vi "Preference_Panel.vi"(0 "Mode":T1) -> ()   [LabVIEW 2010]
uses:
  Anemometry Sub Vis/Controls/Server_Comms.ctl
  Anemometry Sub Vis/Controls/Preference_Mode.ctl
  Anemometry Sub Vis/Controls/Overhead.ctl
  <vilib>/Instr/_visa.llb/VISA Find Search Mode.ctl
  ADAM Client/Sub VIs/ADAM Controls/Calib_type_ADAM.ctl
  ADAM Client/Sub VIs/ADAM Controls/Module_type_ADAM.ctl
  ADAM Client/Sub VIs/ADAM Controls/Ch_description_ADAM.ctl
  ADAM Client/Sub VIs/ADAM Controls/Function_ADAM.ctl
  ADAM Client/Sub VIs/ADAM Controls/Channel_State.ctl
  ADAM Client/Sub VIs/ADAM Controls/Address.ctl
  Anemometry Sub Vis/Globals/Constants_global.vi
  Anemometry Sub Vis/Globals/Preference_global.vi
  Anemometry Sub Vis/Globals/Trav_pos_global.vi
  Anemometry Sub Vis/Globals/Qnet_Globals.vi
  Anemometry Sub Vis/Acquisition/PWA/PWAtasksGLOBAL.vi
  Anemometry Sub Vis/Globals/Dynamic_call_global.ph.vi
panel:
  in  "Post Processing Machine":bool
  in  "Analogue Device Serial No.":string="1188AB4"
  in  "PWA Device Serial No.":string="1187C98"
  in  "ADAM Setup File":u16(ring) items=["Current_Setup.xls"]
  in  "Default Source Establishment Time (s)":dbl=20.0
  out "This Machine's IP Number":string
  in  "Rig Setup":u16(ring) items=["3_x_2_tunnel", "A_Tunnel", "Adam_Sayer_Desk", "ADAM_Server", "Aero_Tunnel", "Alex_Desktop", "B_Tunnel", "Calibration_Tunnel", "Contact_Conductance", "D_Tunnel", "EnFlo_Tunnel", "Frauke_Desktop", "iMac_G5_2", "iMacDuo1", "Matteo's_desktop", "Matteo_PC", "Nick_PC-2", "Paul_Desk-Paul_Desk_Machine", "Paul_Hayden-Desk", "Paul_N_Desk_Machine_2", "Post_Processing_Machine", "PowerBook_G4_1", "PowerBook_G4_2", "Syn_jet_rig", "Tank", "tdf", "Tom_Desk", "Towing_tank", "--New Rig Setup--"]
  in  "Default Traverse Name":u16(ring) items=["A_Tunnel", "Aero_ThroughWall", "Aero_Tunnel", "Angle_Calibrator", "B_Tunnel", "D_Tunnel", "Dummy_Traverse", "EnFlo_Stack", "EnFlo_Tunnel", "EnFlo_Turntable", "Laser_Meas_Traverse", "mohd_setup", "Paul_Desk_Test", "PIV_Traverse", "--New Traverse Setup--"]
  in  "OK":bool
  in  "% Error From First Calib":dbl=10.0 format="%.1f"
  in  "% Error From Previous Calib":dbl=0.5 format="%.1f"
  in  "Qnet Site Root":path=path "/G4_2_HD/Users/paulhayden/Qnet/qnet"
  out "Templates":path=path "/G4_2_HD/Applications (Mac OS 9)/EnFlo Software/Anemometry/Anemometry Sub Vis/Templates"
  in  "Data Folder":path
  out "EnFlo SW Preferences":path=path "/G4_2_HD/Applications (Mac OS 9)/LabVIEW 5.1/EnFlo SW Preferences"
  in  "Tunnel Speed Control":bool
  in  "SMTP server IP address":string
  in  "Abs Press (mbar)":string="Froude:NPL:Atmos_Press"
  in  "Temperature":string="EnFlo Tun:Inlet Heater:Av Temp"
  in  "Server port number":u32=3363
  in  "Server address":string
  in  "LabVIEW Administrators":string[](array[string])=["", "", "", "", "", "", "", "", "", "", "", "", "", "", "", "", "", "", "", ""]
  in  "Server Comms":T2=enum."Do Not Link To Server"
  # "Server Computer Peferences"
  # "Multi Run Preferences"
  # "Warning Levels for Autocalibration Changes"
  # "Email Peferences"
  # "Deg C"
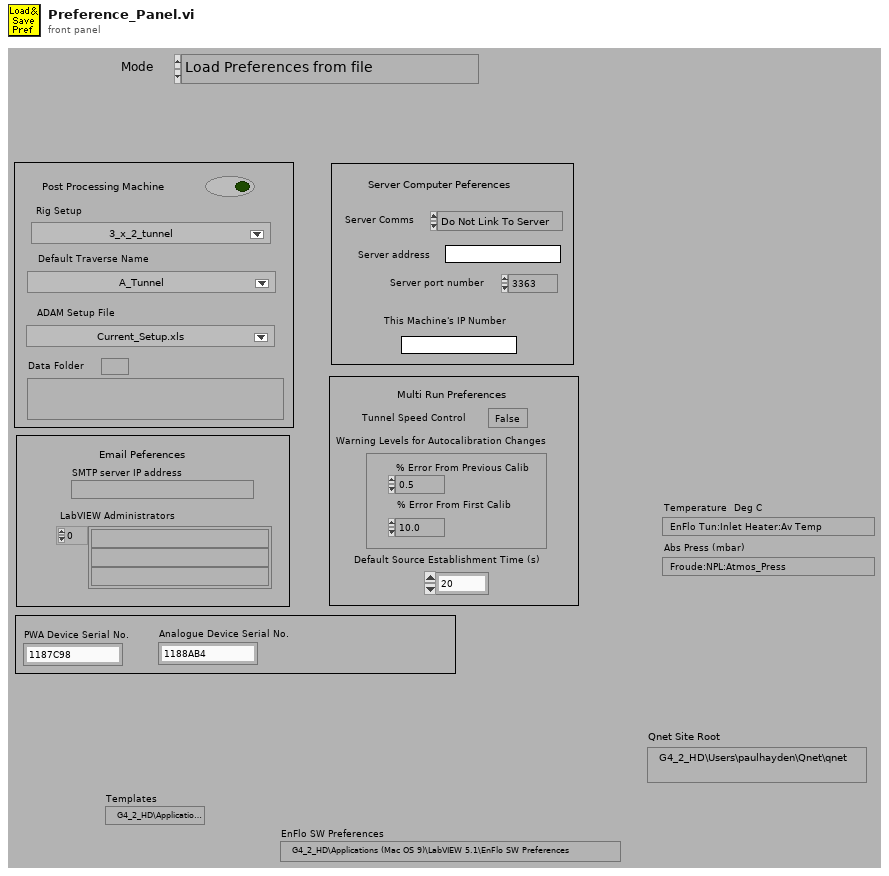
[diagram p1: front panel]
types:
  T1 = typedef "Preference_Mode.ctl" = enum16{"Load Preferences from file", "Save Preferences to file", "Load, Edit then Save"}
  T2 = typedef "Server_Comms.ctl" = enum16{"Server Link Healthy", "Do Not Link To Server"}
  T3 = enum8{"Enabled", "Disabled", "Disabled and Grayed Out"}
  T4 = typedef "Overhead.ctl" = enum16{"Update total times", "Read Current Overhead", "Re Scale totals to 3 hrs", "Initialise totals to 3hr"}
  T5 = typedef "Calib_type_ADAM.ctl" = enum16{"Raw", "Bx + A", "Cx^2 + Bx + A", "Dx^3 + Cx^2 + Bx + A", "In Band", "Hi-Tec Q", "Hi-Tec M_dot", "Text"}
  T6 = typedef "Module_type_ADAM.ctl" = enum16{"4011", "4012", "4013", "4014", "4016", "4017", "4018", "4021", "4050", "4052", "4053", "4060", "4080", "5000", "5017", "5018", "5024", "5051", "5056", "5060", "6060", "Tracker", "WEST", "GILL", "JEM", "VICI", "Vaisala", "DRUCK", "Run VI Named:", "IR2100", "PPT", "Comparator", "VIRTUAL", "Hold Value", "Read A", "Read Ch", "Coded", "Client Info", "Web Client", "X10", "Test"}
  T7 = typedef "Channel_State.ctl" = enum16{"On", "Off", "Always On", "Always Off"}
  T8 = typedef "VISA Find Search Mode.ctl" = u32
  T9 = typedef "Ch_description_ADAM.ctl" = cluster{"Ch Name":string, "Type":T6, "Function":T10, "Ch State":T7, "Calibration type":T5, "A":dbl, "B":dbl, "C":dbl, "D":dbl, "Comments":string, "Address":T11, "String":string, "Duty":u16}
  T10 = typedef "Function_ADAM.ctl" = enum16{"Analogue Input", "Digital Input", "Event counter", "Event rate", "Analogue Output", "Digital Output", "Relay Output"}
  T11 = typedef "Address.ctl" = cluster{"Main":i32, "Ch.":i32, "Sub":i32, "Port Name":string}
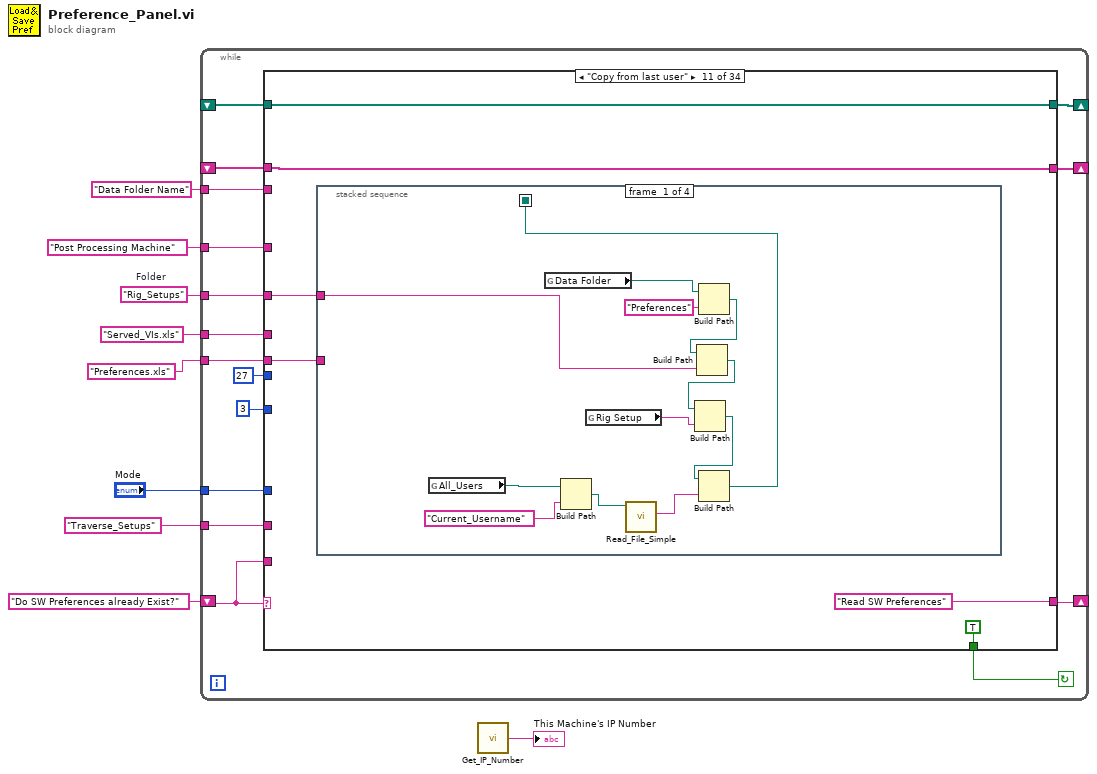
[diagram p0: block diagram]
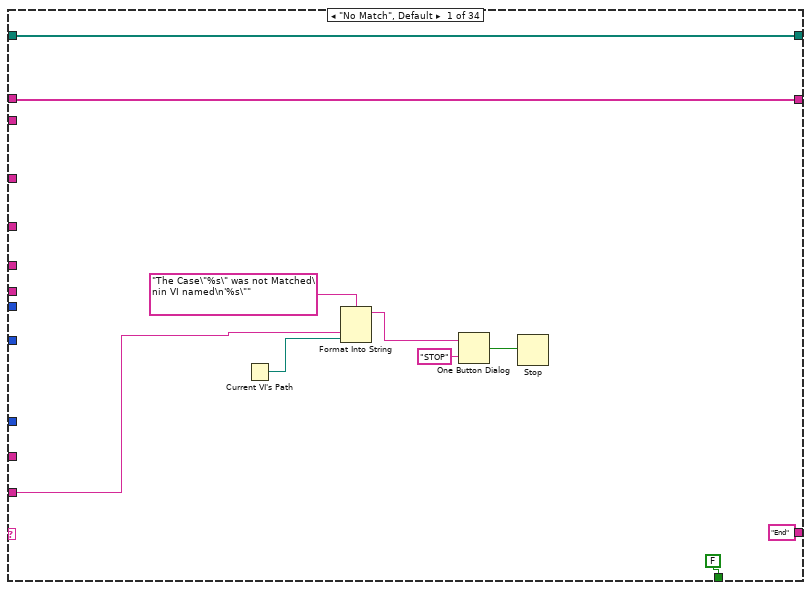
[diagram p2: hidden frame]
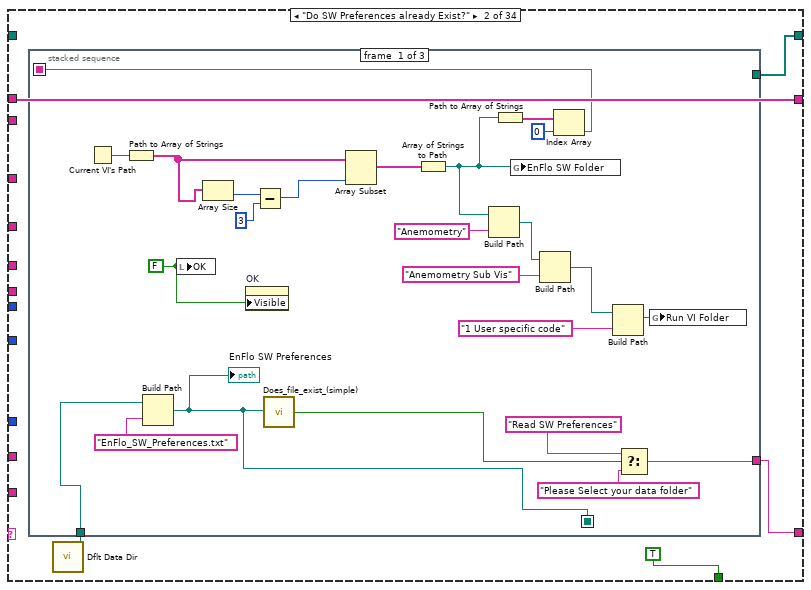
[diagram p3: hidden frame]
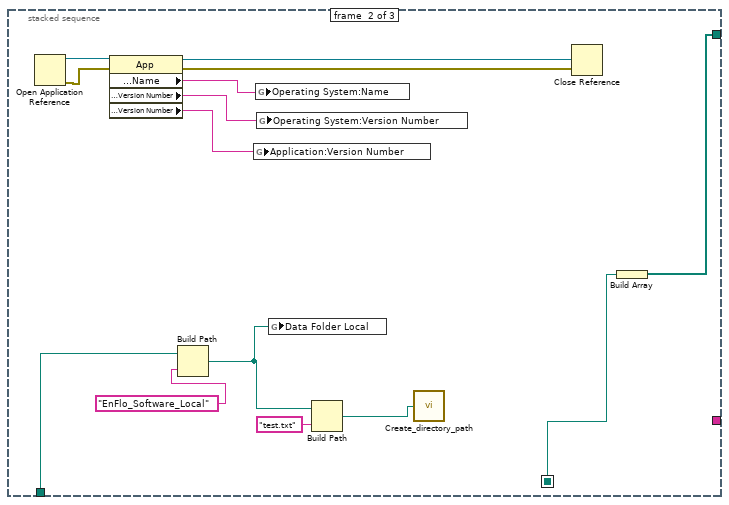
[diagram p4: hidden frame]
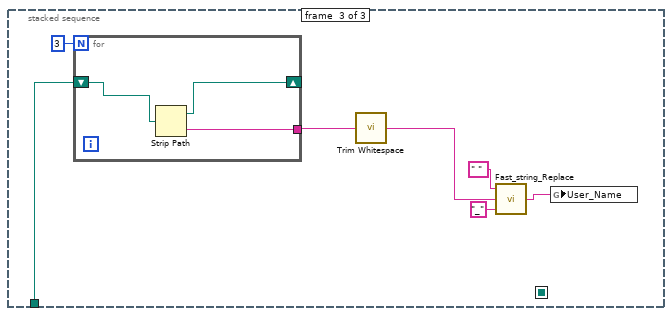
[diagram p5: hidden frame]
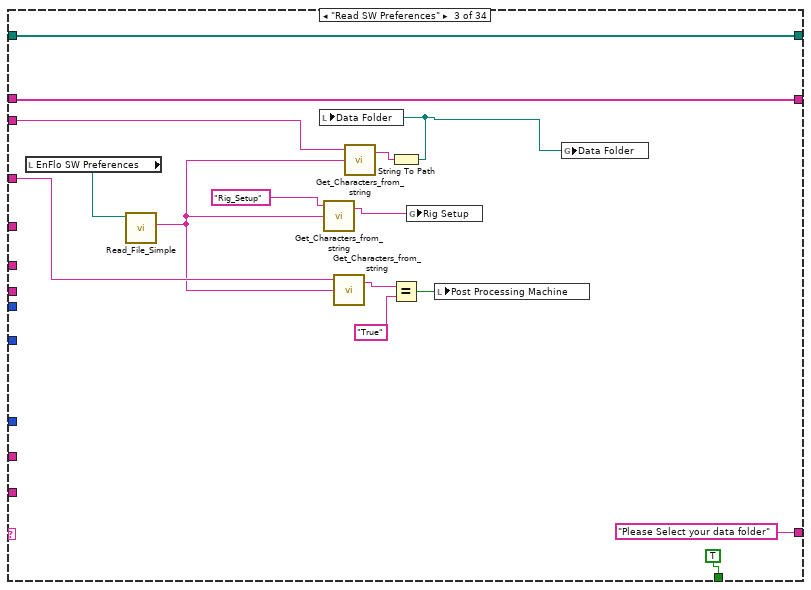
[diagram p6: hidden frame]
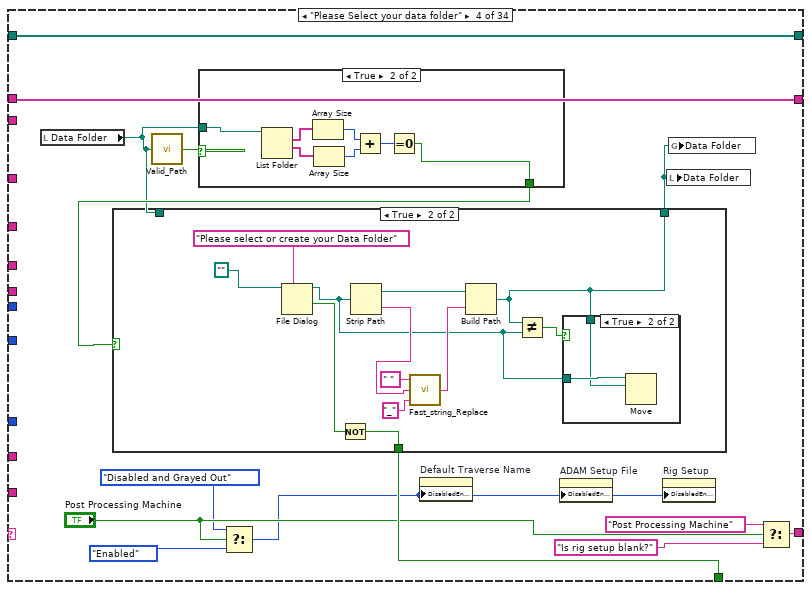
[diagram p7: hidden frame]
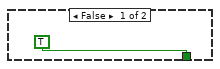
[diagram p8: hidden frame]
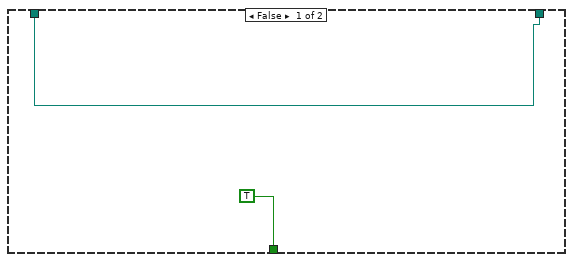
[diagram p9: hidden frame]
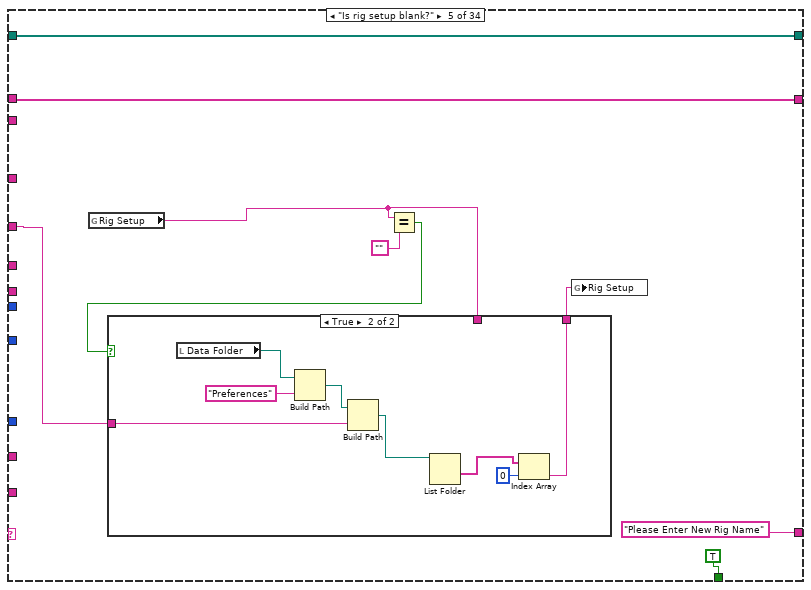
[diagram p11: hidden frame]
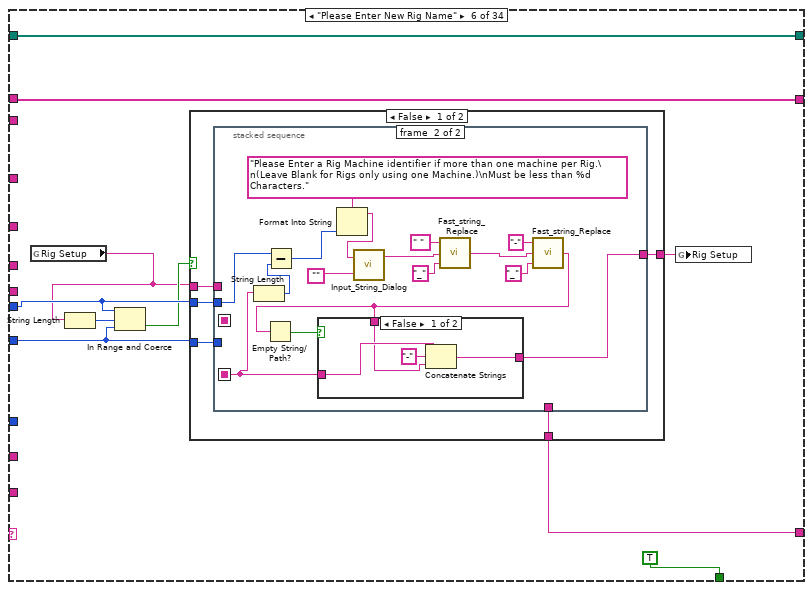
[diagram p13: hidden frame]
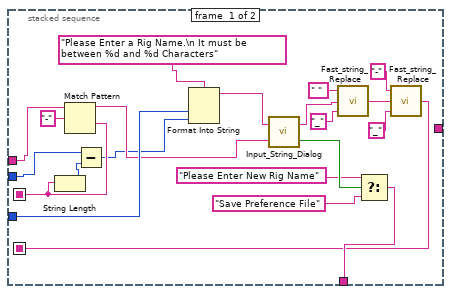
[diagram p14: hidden frame]
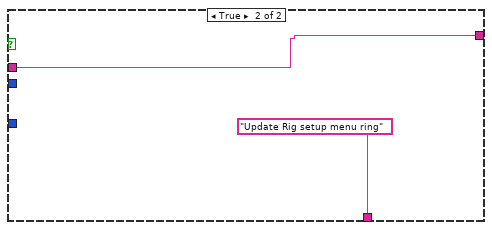
[diagram p16: hidden frame]
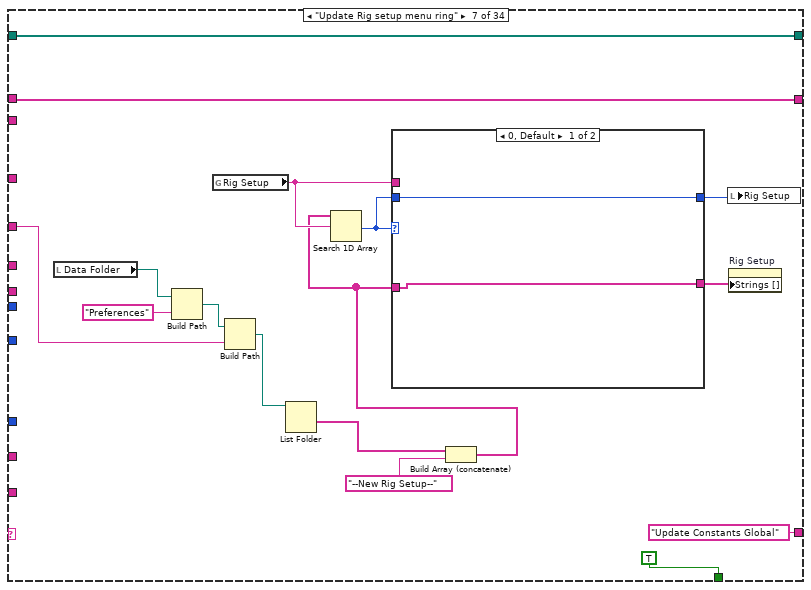
[diagram p17: hidden frame]
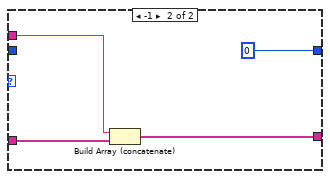
[diagram p18: hidden frame]
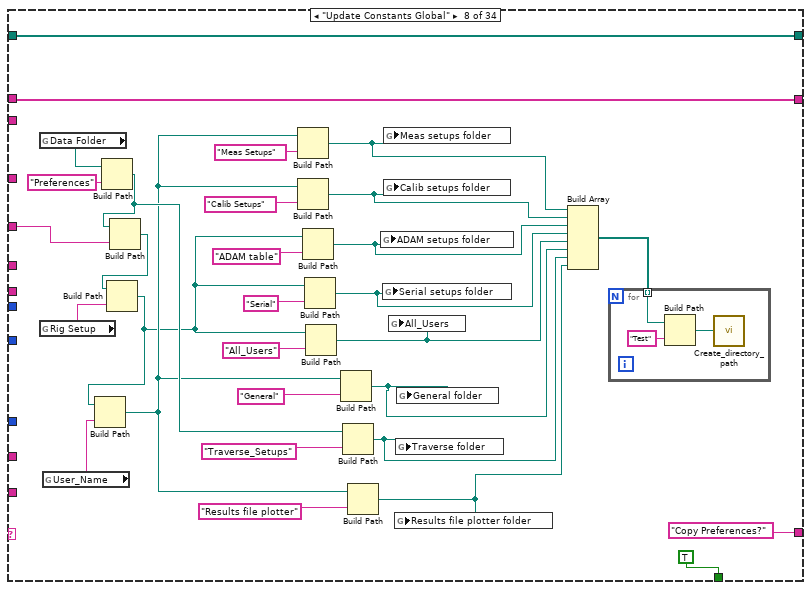
[diagram p19: hidden frame]
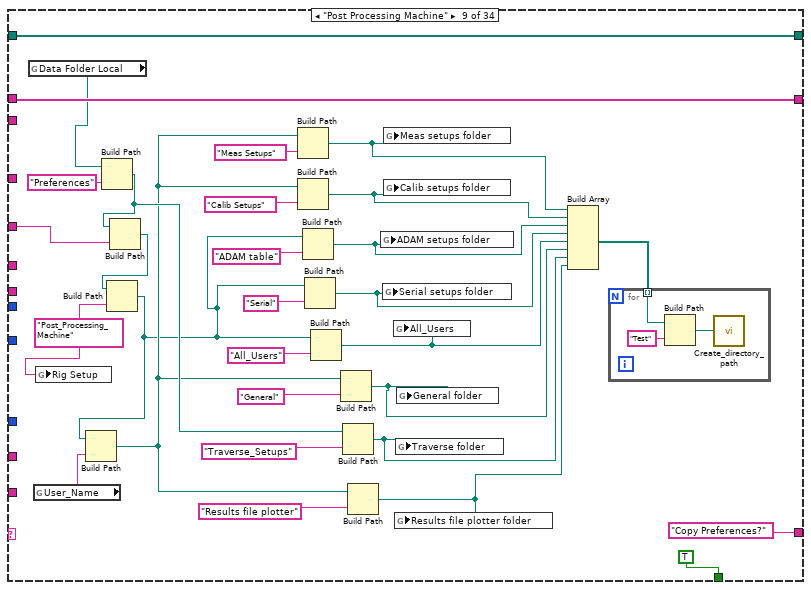
[diagram p20: hidden frame]
diagram:
  w4 = "Rig_Setups"  # Folder
  n1 = while {
    shift-left: _ -> [w22]
    shift-right: [w23] -> _
    shift-left: "Do SW Preferences already Exist?" -> [w21]
    shift-right: [w24] -> _
    tunnel: "Mode" -> [w20]
    tunnel: "Data Folder Name" ("Label for characters") -> [w19]
    tunnel: "Served_VIs.xls" ("Substring") -> [w18]
    tunnel: "Preferences.xls" ("name or relative path") -> [w17]
    tunnel: w4 -> [w14]
    tunnel: "Traverse_Setups" ("name or relative path") -> [w13]
    shift-right: [w12] -> _
    shift-left: _ -> [w11]
    tunnel: "Post Processing Machine" ("Label for characters") -> [w10]
    stop <- w25 continue-if-true
    n2 = case shown="\"Copy from last user\"" w21 {
      tunnel: [FALSE TRUE TRUE w111 TRUE TRUE TRUE TRUE TRUE TRUE TRUE TRUE TRUE TRUE TRUE TRUE TRUE TRUE TRUE TRUE TRUE TRUE TRUE TRUE TRUE TRUE TRUE TRUE TRUE w848 TRUE TRUE TRUE FALSE] -> w25
      tunnel: ["End" w38 "Please Select your data folder" w108 "Please Enter New Rig Name" w166 "Update Constants Global" ("f") "Copy Preferences?" "Copy Preferences?" w312 "Read SW Preferences" "Install Preference files" "Install Adam table files" "Install Adam setup files" "Choose ADAM Setup file" "Preference files continued" "Variable Names" w487 w504 "Please Enter new  Traverse Setup" w579 "Create Traverse setup" ("f") "Check file permission status" w675 w704 w724 w743 w760 "Save Preference File" "Save SW Preferences" w912 w925 "Initialise Globals" "End"] -> w24
      tunnel: [w27 w39 w102 w117 w149 w168 w233 w269 w302 w310 w326 w373 w389 w414 w433 w455 w466 w492 w514 w567 w581 w615 w632 w676 w709 w729 w752 w765 w779 w854 w920 w926 w978 w1038] -> w23
      tunnel: w22 -> [w27 w39 w102 w117 w149 w168 w233 w269 w302 w310 w326 w373 w389 w414 w433 w455 w466 _ w514 w567 w581 w615 w632 w676 w709 w729 w752 w765 w779 w854 w920 w926 w978 w1038]
      tunnel: w21 -> [w30 _ _ _ _ _ _ _ _ _ _ _ _ _ _ _ _ _ _ _ _ _ _ _ _ _ _ _ _ _ _ _ _ _]
      tunnel: w20 -> [_ _ _ _ _ _ _ _ _ _ _ _ _ _ _ _ _ w486 _ _ _ _ _ w674 _ _ _ _ _ w849 _ _ _ _]
      tunnel: w19 -> [_ _ w98 _ _ _ _ _ _ _ _ _ _ _ _ _ _ _ _ _ _ _ _ _ _ _ _ _ _ _ w911 _ _ _]
      tunnel: w18 -> [_ _ _ _ _ _ _ _ _ _ _ _ w383 _ _ _ _ _ _ _ _ _ _ _ _ _ _ _ _ _ _ _ w970 _]
      tunnel: w17 -> [_ _ _ _ _ _ _ _ _ w307 w324 _ _ _ _ _ _ _ w510 _ _ _ _ _ _ _ _ _ _ w846 _ _ _ _]
      tunnel: 3 ("lower limit") -> [_ _ _ _ _ w165 _ _ _ _ _ _ _ _ _ _ _ _ _ _ w578 _ _ _ _ _ _ _ _ _ _ _ _ _]
      tunnel: 27 ("upper limit") -> [_ _ _ _ _ w164 _ _ _ _ _ _ _ _ _ _ _ _ _ _ w577 _ _ _ _ _ _ _ _ _ _ _ _ _]
      tunnel: w14 -> [_ _ _ _ w146 _ w221 w249 w282 _ w323 _ _ _ _ _ _ _ _ _ _ _ _ _ _ _ _ _ _ _ _ _ _ _]
      tunnel: w13 -> [_ _ _ _ _ _ _ _ _ _ _ _ _ _ _ _ _ _ _ w565 _ w602 _ _ _ _ _ _ w778 _ _ _ _ _]
      tunnel: [w26 w36 w94 w112 w143 w160 w219 w246 w281 w311 w327 w364 w379 w407 w430 w441 w457 w479 w508 w564 w573 w601 w628 path[] [] w701 w721 w746 w763 w777 w844 w908 w924 w969 w1035] -> w12
      tunnel: w11 -> [w26 _ w94 w112 w143 w160 w219 w246 w281 w311 w327 w363 w381 w407 w431 w441 w459 w479 w509 w564 w573 w601 w629 w673 w701 w721 w746 w763 w777 w844 w908 w924 w969 w1035]
      tunnel: w10 -> [_ _ w93 _ _ _ _ _ _ _ _ _ _ _ _ _ _ _ _ _ _ _ _ _ _ _ _ _ _ _ w902 _ _ _]
      frame "No Match", Default {
        n3 = Current VI's Path() -> (path=w35:path)
        n4 = Format Into String(format string="The Case\"%s\" was not Matched\nin VI named\n'%s\"" ("Format String"), w30, w35) -> (resulting string=w32:string)  [unwired: 2 in, 1 out]
        n5 = One Button Dialog(message=w32, button name ("OK")="STOP") -> (true=w34:bool)
        n6 = Stop(stop? (T)=w34) -> ()
      }
      frame "Do SW Preferences already Exist?" {
        n7 = call <vilib>:"Dflt Data Dir.vi"() -> ("App:Default Data Directory"=w37:path)
        n8 = stacked-sequence {
          seq-local: [w44 _ _] -> [_ _ _]
          seq-local: [w42 _ _] -> [_ w70 _]
          tunnel: [w48 _ _] -> w38
          tunnel: w37 -> [w43 w68 w84]
          tunnel: [_ w71 _] -> w36
          frame #0 {
            w41 = FALSE ("OK")
            n9 = Current VI's Path() -> (path=w62:path)
            n10 = Path to Array of Strings(0:w62) -> (2:w59:string[])  [unwired: 1 out]
            n11 = Build Path(base path=w43, name or relative path="EnFlo_SW_Preferences.txt") -> (appended path=w42:path)
            "EnFlo SW Preferences" <- w42
            n12 = local write "OK"(w41) -> ()
            n13 = Array Size(array=w59) -> (size(s)=w61:i32)
            n14 = property on="OK" class="Bool (strict)"("Visible"=w41) -> ()  [unwired: 2 in, 2 out]
            n15 = Subtract(x=w61, y=3) -> (x-y=w57:i32)
            n16 = call "Does_file_exist_(simple).vi"("Pathname"=w42) -> ("exists?"=w63:bool)
            n17 = Array Subset(array=w59, length=w57) -> (w58:string[])  [unwired: 1 in]
            n18 = Array of Strings to Path(0:w58) -> (2:w45:path)  [unwired: 1 out]
            n19 = Build Path(base path=w45, name or relative path="Anemometry") -> (appended path=w54:path)
            n20 = Path to Array of Strings(0:w45) -> (2:w46:string[])  [unwired: 1 out]
            n21 = global write "Constants_global.vi" "EnFlo SW Folder"(w45) -> ()
            n22 = Build Path(base path=w54, name or relative path="Anemometry Sub Vis") -> (appended path=w52:path)
            n23 = Index Array(array=w46, index=0) -> (element=w44:string)
            n24 = Build Path(base path=w52, name or relative path="1 User specific code") -> (appended path=w51:path)
            n25 = Select(t="Read SW Preferences", s=w63, f="Please Select your data folder") -> (s? t:f=w48:string)
            n26 = global write "Constants_global.vi" "Run VI Folder"(w51) -> ()
          }
          frame #1 {
            n27 = Open Application Reference() -> (0:w75:errorcluster, 3:w78:refnum<vi>)  [unwired: 1 in, 3 out]
            n28 = property class="App"(reference=w78, error in=w75) -> (reference out=w77:refnum<vi>, error out=w76:errorcluster, "Operating System:Name"=w72:string, "Operating System:Version Number"=w74:string, "Application:Version Number"=w73:string)
            n29 = Build Path(base path=w68, name or relative path="EnFlo_Software_Local" ("element")) -> (appended path=w67:path)
            n30 = global write "Preference_global.vi" "Application:Version Number"(w73) -> ()
            n31 = global write "Preference_global.vi" "Operating System:Name"(w72) -> ()
            n32 = global write "Preference_global.vi" "Operating System:Version Number"(w74) -> ()
            n33 = global write "Constants_global.vi" "Data Folder Local"(w67) -> ()
            n34 = Build Path(base path=w67, name or relative path="test.txt") -> (appended path=w65:path)
            n35 = call "Create_directory_path.vi"("Path name"=w65) -> ()  [unwired: 1 out]
            n36 = Close Reference(reference=w77, error in (no error)=w76) -> ()  [unwired: 1 out]
            n37 = Build Array(w70) -> (w71:path[])
          }
          frame #2 {
            n38 = for {
              N: 3 -> [_]
              shift-right: [w88] -> _
              shift-left: w84 -> [w87]
              tunnel: [w86] -> w80
              n39 = Strip Path(path=w87) -> (stripped path=w88:path, name=w86:string)
            }
            n40 = call <vilib>:"Trim Whitespace.vi"("string"=w80) -> ("trimmed string"=w79:string)  [unwired: 1 in]
            n41 = call "Fast_string_Replace.vi"("Replace match with:"="_", "Input String"=w79, "regular expression"=" ") -> ("Output String"=w81:string)  [unwired: 1 in, 1 out]
            n42 = global write "Preference_global.vi" "User_Name"(w81) -> ()
          }
        }
      }
      frame "Read SW Preferences" {
        n43 = local read "EnFlo SW Preferences"() -> (w101:path)
        n44 = call "Read_File_Simple.vi"("Filename"=w101) -> ("string"=w92:string)  [unwired: 2 in, 7 out]
        n45 = call "Get_Characters_from_string.vi"("Input string"=w92, "Variable name"="Rig_Setup" ("Label for characters")) -> ("Value"=w95:string)  [unwired: 1 in, 1 out]
        n46 = call "Get_Characters_from_string.vi"("Input string"=w92, "Variable name"=w93) -> ("Value"=w91:string)  [unwired: 1 in, 1 out]
        n47 = call "Get_Characters_from_string.vi"("Input string"=w92, "Variable name"=w98) -> ("Value"=w99:string)  [unwired: 1 in, 1 out]
        n48 = String To Path(string=w99) -> (path=w97:path)
        n49 = local write "Data Folder"(w97) -> ()
        n50 = Equal?(x=w91, y="True") -> (x = y?=w89:bool)
        n51 = global write "Preference_global.vi" "Rig Setup"(w95) -> ()
        n52 = local write "Post Processing Machine"(w89) -> ()
        n53 = global write "Constants_global.vi" "Data Folder"(w97) -> ()
      }
      frame "Please Select your data folder" {
        n54 = local read "Data Folder"() -> (w113:path)
        n55 = call "Valid_Path.vi"("Filename"=w113) -> ("Valid Path?"=w115:bool)
        n56 = case shown="True" w115 {
          tunnel: [TRUE ("status") w119] -> w114
          tunnel: w113 -> [_ w125]
          frame False {
          }
          frame True {
            n57 = List Folder(path=w125) -> (filenames=w123:string[], folder names=w124:string[])  [unwired: 1 in, 4 out]
            n58 = Array Size(array=w123) -> (size(s)=w121:i32)
            n59 = Array Size(array=w124) -> (size(s)=w122:i32)
            n60 = Add(x=w121, y=w122) -> (x+y=w120:i32)
            n61 = Equal To 0?(x=w120) -> (x = 0?=w119:bool)
          }
        }
        n62 = case shown="True" w114 {
          tunnel: [w127 w130] -> w116
          tunnel: w113 -> [w127 _]
          tunnel: [TRUE w128] -> w111
          frame False {
          }
          frame True {
            n63 = File Dialog(7:"Please select or create your Data Folder" ("prompt"), 11:path "") -> (1:w129:bool, 3:w131:path)  [unwired: 1 in, 6 out]
            n64 = Not(x=w129) -> (.not. x?=w128:bool)
            n65 = Strip Path(path=w131) -> (stripped path=w135:path, name=w134:string)
            n66 = call "Fast_string_Replace.vi"("Replace match with:"="_", "Input String"=w134, "regular expression"=" ") -> ("Output String"=w133:string)  [unwired: 2 out]
            n67 = Build Path(base path=w135, name or relative path=w133) -> (appended path=w130:path)
            n68 = Not Equal?(x=w130, y=w131) -> (x != y?=w132:bool)
            n69 = case shown="True" w132 {
              tunnel: w131 -> [_ w141]
              tunnel: w130 -> [_ w140]
              frame False {
              }
              frame True {
                n70 = Move(source path=w141, 10:w140) -> ()  [unwired: 1 in, 5 out]
              }
            }
          }
        }
        n71 = Select(t=T3."Disabled and Grayed Out" ("Disabled"), s="Post Processing Machine", f=T3."Enabled" ("Disabled")) -> (s? t:f=w104:T3)
        n72 = property on="Default Traverse Name" class="Ring (strict)"("DisabledEnum"=w104) -> ()  [unwired: 2 in, 2 out]
        n73 = property on="ADAM Setup File" class="Ring (strict)"("DisabledEnum"=w104) -> ()  [unwired: 2 in, 2 out]
        n74 = property on="Rig Setup" class="Ring (strict)"("DisabledEnum"=w104) -> ()  [unwired: 2 in, 2 out]
        n75 = local write "Data Folder"(w116) -> ()
        n76 = global write "Constants_global.vi" "Data Folder"(w116) -> ()
        n77 = Select(t="Post Processing Machine", s="Post Processing Machine", f="Is rig setup blank?") -> (s? t:f=w108:string)
      }
      frame "Is rig setup blank?" {
        n78 = global read "Preference_global.vi" "Rig Setup"() -> (w144:string)
        n79 = Equal?(x=w144, y="") -> (x = y?=w147:bool)
        n80 = case shown="True" w147 {
          tunnel: w146 -> [_ w155]
          tunnel: [w151 w152] -> w145
          tunnel: w144 -> [w151 _]
          frame False {
          }
          frame True {
            n81 = local read "Data Folder"() -> (w158:path)
            n82 = Build Path(base path=w158, name or relative path="Preferences") -> (appended path=w157:path)
            n83 = Build Path(base path=w157, name or relative path=w155) -> (appended path=w156:path)
            n84 = List Folder(path=w156) -> (folder names=w153:string[])  [unwired: 1 in, 5 out]
            n85 = Index Array(array=w153, index=0) -> (element=w152:string)
          }
        }
        n86 = global write "Preference_global.vi" "Rig Setup"(w145) -> ()
      }
      frame "Please Enter New Rig Name" {
        n87 = global read "Preference_global.vi" "Rig Setup"() -> (w162:string)
        n88 = String Length(string=w162) -> (length=w167:i32)
        n89 = In Range and Coerce(upper limit=w164, x=w167, lower limit=w165) -> (In Range?=w163:bool)  [unwired: 1 out]
        n90 = case shown="False" w163 {
          tunnel: w162 -> [w174 w217]
          tunnel: [w170 "Update Rig setup menu ring"] -> w166
          tunnel: [w171 w217] -> w161
          tunnel: w165 -> [w173 _]
          tunnel: w164 -> [w172 _]
          frame False {
            n91 = stacked-sequence {
              seq-local: [w175 _] -> [_ w200]
              seq-local: [w182 _] -> [_ _]
              tunnel: w174 -> [w184 _]
              tunnel: w173 -> [w195 _]
              tunnel: w172 -> [w181 w198]
              tunnel: [_ w203] -> w171
              tunnel: [w187 _] -> w170
              frame #0 {
                n92 = Match Pattern(string=w184, regular expression="-") -> (before substring=w183:string, after substring=w182:string)  [unwired: 3 out]
                n93 = String Length(string=w182) -> (length=w180:i32)
                n94 = Subtract(x=w181, y=w180) -> (x-y=w179:i32)
                n95 = Format Into String(format string="Please Enter a Rig Name.\n It must be between %d and %d Characters" ("Message to user"), w195, w179) -> (resulting string=w194:string)  [unwired: 2 in, 1 out]
                n96 = call "Input_String_Dialog.vi"("Value"=w183, "Message to user"=w194) -> ("Ok Out"=w190:bool, "Output string"=w191:string)
                n97 = call "Fast_string_Replace.vi"("Replace match with:"="_", "Input String"=w191, "regular expression"=" ") -> ("Output String"=w176:string)  [unwired: 2 out]
                n98 = Select(t="Please Enter New Rig Name", s=w190, f="Save Preference File") -> (s? t:f=w187:string)
                n99 = call "Fast_string_Replace.vi"("Replace match with:"="_", "Input String"=w176, "regular expression"="-") -> ("Output String"=w175:string)  [unwired: 2 out]
              }
              frame #1 {
                n100 = String Length(string=w200) -> (length=w199:i32)
                n101 = Subtract(x=w198, y=w199) -> (x-y=w197:i32)
                n102 = Format Into String(format string="Please Enter a Rig Machine identifier if more than one machine per Rig.\n(Leave Blank for Rigs only using one Machine.)\nMust be less than %d Characters." ("Message to user"), w197) -> (resulting string=w196:string)  [unwired: 2 in, 1 out]
                n103 = call "Input_String_Dialog.vi"("Value"="", "Message to user"=w196) -> ("Output string"=w209:string)  [unwired: 1 out]
                n104 = call "Fast_string_Replace.vi"("Replace match with:"="_", "Input String"=w209, "regular expression"=" ") -> ("Output String"=w205:string)  [unwired: 2 out]
                n105 = call "Fast_string_Replace.vi"("Replace match with:"="_", "Input String"=w205, "regular expression"="-") -> ("Output String"=w202:string)  [unwired: 2 out]
                n106 = Empty String/Path?(string/path=w202) -> (empty?=w204:bool)
                n107 = case shown="False" w204 {
                  tunnel: [w212 w216] -> w203
                  tunnel: w200 -> [w215 w216]
                  tunnel: w202 -> [w213 _]
                  frame False {
                    n108 = Concatenate Strings(w215, "-" ("string"), w213) -> (w212:string)
                  }
                  frame True {
                  }
                }
              }
            }
          }
          frame True {
          }
        }
        n109 = global write "Preference_global.vi" "Rig Setup"(w161) -> ()
      }
      frame "Update Rig setup menu ring" {
        n110 = local read "Data Folder"() -> (w224:path)
        n111 = Build Path(base path=w224, name or relative path="Preferences") -> (appended path=w223:path)
        n112 = global read "Preference_global.vi" "Rig Setup"() -> (w230:string)
        n113 = Build Path(base path=w223, name or relative path=w221) -> (appended path=w222:path)
        n114 = List Folder(path=w222) -> (folder names=w220:string[])  [unwired: 1 in, 5 out]
        n115 = Build Array (concatenate)(w220, "--New Rig Setup--") -> (w226:string[])
        n116 = Search 1D Array(1D array=w226, element=w230) -> (index of element=w229:i32)  [unwired: 1 out]
        n117 = case shown="0, Default" w229 {
          tunnel: [w236 0] -> w232
          tunnel: w226 -> [w235 w239]
          tunnel: w230 -> [_ w238]
          tunnel: w229 -> [w236 _]
          tunnel: [w235 w237] -> w228
          frame 0, Default {
          }
          frame -1 {
            n118 = Build Array (concatenate)(w238, w239) -> (w237:string[])
          }
        }
        n119 = local write "Rig Setup"(w232) -> ()
        n120 = property on="Rig Setup" class="Ring (strict)"("Strings []"=w228) -> ()  [unwired: 2 in, 2 out]
      }
      frame "Update Constants Global" {
        n121 = global read "Constants_global.vi" "Data Folder"() -> (w247:path)
        n122 = global read "Preference_global.vi" "Rig Setup"() -> (w248:string)
        n123 = global read "Preference_global.vi" "User_Name"() -> (w245:string)
        n124 = Build Path(base path=w247, name or relative path="Preferences") -> (appended path=w250:path)
        n125 = Build Path(base path=w250, name or relative path=w249) -> (appended path=w251:path)
        n126 = Build Path(base path=w251, name or relative path=w248) -> (appended path=w241:path)
        n127 = Build Path(base path=w241, name or relative path=w245) -> (appended path=w244:path)
        n128 = Build Path(base path=w244, name or relative path="Meas Setups") -> (appended path=w261:path)
        n129 = Build Path(base path=w244, name or relative path="Calib Setups") -> (appended path=w260:path)
        n130 = Build Path(base path=w241, name or relative path="ADAM table") -> (appended path=w259:path)
        n131 = Build Path(base path=w241, name or relative path="Serial") -> (appended path=w258:path)
        n132 = Build Path(base path=w241, name or relative path="All_Users") -> (appended path=w242:path)
        n133 = Build Path(base path=w244, name or relative path="General") -> (appended path=w257:path)
        n134 = Build Path(base path=w250, name or relative path="Traverse_Setups") -> (appended path=w256:path)
        n135 = Build Path(base path=w244, name or relative path="Results file plotter") -> (appended path=w252:path)
        n136 = global write "Constants_global.vi" "ADAM setups folder"(w259) -> ()
        n137 = global write "Constants_global.vi" "Serial setups folder"(w258) -> ()
        n138 = global write "Constants_global.vi" "Meas setups folder"(w261) -> ()
        n139 = global write "Constants_global.vi" "Calib setups folder"(w260) -> ()
        n140 = global write "Constants_global.vi" "All_Users"(w242) -> ()
        n141 = global write "Constants_global.vi" "Results file plotter folder"(w252) -> ()
        n142 = global write "Constants_global.vi" "Traverse folder"(w256) -> ()
        n143 = global write "Constants_global.vi" "General folder"(w257) -> ()
        n144 = Build Array(w261, w260, w259, w258, w242, w257, w256, w252) -> (w255:path[])
        n145 = for {
          tunnel: w255 -> [w273] mode=indexing
          n146 = Build Path(base path=w273, name or relative path="Test") -> (appended path=w271:path)
          n147 = call "Create_directory_path.vi"("Path name"=w271) -> ()  [unwired: 1 out]
        }
      }
      frame "Post Processing Machine" {
        w279 = "Post_Processing_Machine" ("Rig Setup")
        n148 = global read "Constants_global.vi" "Data Folder Local"() -> (w280:path)
        n149 = global read "Preference_global.vi" "User_Name"() -> (w278:string)
        n150 = global write "Preference_global.vi" "Rig Setup"(w279) -> ()
        n151 = Build Path(base path=w280, name or relative path="Preferences") -> (appended path=w283:path)
        n152 = Build Path(base path=w283, name or relative path=w282) -> (appended path=w284:path)
        n153 = Build Path(base path=w284, name or relative path=w279) -> (appended path=w274:path)
        n154 = Build Path(base path=w274, name or relative path=w278) -> (appended path=w277:path)
        n155 = Build Path(base path=w277, name or relative path="Meas Setups") -> (appended path=w294:path)
        n156 = Build Path(base path=w277, name or relative path="Calib Setups") -> (appended path=w293:path)
        n157 = Build Path(base path=w274, name or relative path="ADAM table") -> (appended path=w292:path)
        n158 = Build Path(base path=w274, name or relative path="Serial") -> (appended path=w291:path)
        n159 = Build Path(base path=w274, name or relative path="All_Users") -> (appended path=w275:path)
        n160 = Build Path(base path=w277, name or relative path="General") -> (appended path=w290:path)
        n161 = Build Path(base path=w283, name or relative path="Traverse_Setups") -> (appended path=w289:path)
        n162 = Build Path(base path=w277, name or relative path="Results file plotter") -> (appended path=w285:path)
        n163 = global write "Constants_global.vi" "ADAM setups folder"(w292) -> ()
        n164 = global write "Constants_global.vi" "Serial setups folder"(w291) -> ()
        n165 = global write "Constants_global.vi" "Meas setups folder"(w294) -> ()
        n166 = global write "Constants_global.vi" "Calib setups folder"(w293) -> ()
        n167 = global write "Constants_global.vi" "All_Users"(w275) -> ()
        n168 = global write "Constants_global.vi" "Results file plotter folder"(w285) -> ()
        n169 = global write "Constants_global.vi" "Traverse folder"(w289) -> ()
        n170 = global write "Constants_global.vi" "General folder"(w290) -> ()
        n171 = Build Array(w294, w293, w292, w291, w275, w290, w289, w285) -> (w288:path[])
        n172 = for {
          tunnel: w288 -> [w306] mode=indexing
          n173 = Build Path(base path=w306, name or relative path="Test") -> (appended path=w304:path)
          n174 = call "Create_directory_path.vi"("Path name"=w304) -> ()  [unwired: 1 out]
        }
      }
      frame "Copy Preferences?" {
        n175 = global read "Constants_global.vi" "General folder"() -> (w317:path)
        n176 = Build Path(base path=w317, name or relative path=w307) -> (appended path=w316:path)
        n177 = call <vilib>:"Check if File or Folder Exists.vi"("path"=w316) -> ("file or folder exists?"=w309:bool)  [unwired: 1 in, 9 out]
        n178 = case shown="False" w309 {
          tunnel: [w318 TRUE ("Error?")] -> w308
          frame False {
            n179 = global read "Constants_global.vi" "All_Users"() -> (w320:path)
            n180 = Build Path(base path=w320, name or relative path="Current_Username") -> (appended path=w321:path)
            n181 = call "Read_File_Simple.vi"("Filename"=w321) -> ("Error?"=w318:bool)  [unwired: 4 in, 5 out]
          }
          frame True {
          }
        }
        n182 = Select(t="Install Generic Meas Setup file", s=w308, f="Copy from last user") -> (s? t:f=w312:string)
      }
      frame "Copy from last user" {
        n183 = stacked-sequence {
          seq-local: [w333 _ _ _] -> [_ w342 w348 w355]
          tunnel: w324 -> [_ w341 _ _]
          tunnel: w323 -> [w329 _ _ _]
          frame #0 {
            n184 = global read "Constants_global.vi" "All_Users"() -> (w338:path)
            n185 = global read "Constants_global.vi" "Data Folder"() -> (w332:path)
            n186 = Build Path(base path=w338, name or relative path="Current_Username") -> (appended path=w336:path)
            n187 = global read "Preference_global.vi" "Rig Setup"() -> (w340:string)
            n188 = call "Read_File_Simple.vi"("Filename"=w336) -> ("string"=w335:string)  [unwired: 4 in, 5 out]
            n189 = Build Path(base path=w332, name or relative path="Preferences") -> (appended path=w331:path)
            n190 = Build Path(base path=w331, name or relative path=w329) -> (appended path=w330:path)
            n191 = Build Path(base path=w330, name or relative path=w340) -> (appended path=w334:path)
            n192 = Build Path(base path=w334, name or relative path=w335) -> (appended path=w333:path)
          }
          frame #1 {
            n193 = global read "Constants_global.vi" "General folder"() -> (w344:path)
            n194 = Build Path(base path=w344, name or relative path=w341) -> (appended path=w343:path)
            n195 = Build Path(base path=w342, name or relative path="General") -> (appended path=w346:path)
            n196 = Build Path(base path=w346, name or relative path=w341) -> (appended path=w345:path)
            n197 = Copy(10:w343, 11:w345) -> ()  [unwired: 3 in, 3 out]
          }
          frame #2 {
            w351 = "Current_Setup.xls"
            n198 = Build Path(base path=w348, name or relative path="Meas Setups") -> (appended path=w352:path)
            n199 = global read "Constants_global.vi" "Meas setups folder"() -> (w353:path)
            n200 = Build Path(base path=w352, name or relative path=w351) -> (appended path=w350:path)
            n201 = Build Path(base path=w353, name or relative path=w351) -> (appended path=w349:path)
            n202 = Copy(10:w349, 11:w350) -> ()  [unwired: 3 in, 3 out]
          }
          frame #3 {
            w358 = "Current_Setup.xls"
            n203 = Build Path(base path=w355, name or relative path="Calib Setups") -> (appended path=w359:path)
            n204 = global read "Constants_global.vi" "Calib setups folder"() -> (w360:path)
            n205 = Build Path(base path=w359, name or relative path=w358) -> (appended path=w357:path)
            n206 = Build Path(base path=w360, name or relative path=w358) -> (appended path=w356:path)
            n207 = Copy(10:w356, 11:w357) -> ()  [unwired: 3 in, 3 out]
          }
        }
      }
      frame "Install Generic Meas Setup file" {
        n208 = global read "Constants_global.vi" "Run VI Folder"() -> (w372:path)
        n209 = global read "Constants_global.vi" "Meas setups folder"() -> (w369:path)
        n210 = Strip Path(path=w372) -> (stripped path=w370:path)  [unwired: 1 out]
        n211 = Build Path(base path=w369, name or relative path="Current_Setup.xls") -> (appended path=w362:path)
        n212 = Build Path(base path=w370, name or relative path="Templates") -> (appended path=w366:path)
        "Templates" <- w366
        n213 = call "Does_file_exist_(simple).vi"("Pathname"=w362) -> ("exists?"=w367:bool)
        n214 = case shown="False" w367 {
          tunnel: w362 -> [w378 _]
          tunnel: w366 -> [w376 _]
          frame False {
            n215 = Build Path(base path=w376, name or relative path="Measurement Setup.xls") -> (appended path=w375:path)
            n216 = Copy(10:w378, 11:w375) -> ()  [unwired: 1 in, 5 out]
          }
          frame True {
          }
        }
        n217 = Build Array (concatenate)(w363, w362) -> (w364:path[])
      }
      frame "Install Preference files" {
        n218 = global read "Constants_global.vi" "General folder"() -> (w386:path)
        n219 = Build Array("Preferences.xls" ("Substring"), w383, "Month_Names.xls" ("name or relative path"), "LDA_Configuration.xls") -> (w388:string[])
        n220 = for {
          tunnel: w388 -> [w392] mode=indexing
          tunnel: w386 -> [w393]
          tunnel: [w391] -> w380 mode=indexing
          n221 = Build Path(base path=w393, name or relative path=w392) -> (appended path=w391:path)
          n222 = call "Does_file_exist_(simple).vi"("Pathname"=w391) -> ("exists?"=w394:bool)
          n223 = case shown="False" w394 {
            tunnel: w391 -> [w398 _]
            tunnel: w392 -> [w395 _]
            frame False {
              n224 = local read "Templates"() -> (w396:path)
              n225 = Build Path(base path=w396, name or relative path=w395) -> (appended path=w397:path)
              n226 = Copy(10:w398, 11:w397) -> ()  [unwired: 1 in, 5 out]
            }
            frame True {
            }
          }
        }
        n227 = Build Array (concatenate)(w381, w380) -> (w379:path[])
      }
      frame "Install Adam table files" {
        w403 = "Current_Setup.xls"
        n228 = global read "Constants_global.vi" "ADAM setups folder"() -> (w405:path)
        n229 = Build Path(base path=w405, name or relative path=w403) -> (appended path=w406:path)
        n230 = Build Path(base path=w405, name or relative path="Setup_Files") -> (appended path=w401:path)
        n231 = Build Array("Hi_Tec_Calibs.xls" ("name or relative path"), "A_Tunnel DB setup.xls" ("Substring"), "EnFlo_Tunnel DB setup.xls", "Aero_Tunnel DB setup.xls" ("name or relative path"), "D_Tunnel DB setup.xls") -> (w413:string[])
        n232 = Build Path(base path=w401, name or relative path=w403) -> (appended path=w400:path)
        n233 = for {
          tunnel: w413 -> [w417] mode=indexing
          tunnel: w405 -> [w418]
          n234 = Build Path(base path=w418, name or relative path=w417) -> (appended path=w416:path)
          n235 = call "Does_file_exist_(simple).vi"("Pathname"=w416) -> ("exists?"=w419:bool)
          n236 = case shown="False" w419 {
            tunnel: w416 -> [w423 _]
            tunnel: w417 -> [w420 _]
            frame False {
              n237 = local read "Templates"() -> (w421:path)
              n238 = Build Path(base path=w421, name or relative path=w420) -> (appended path=w422:path)
              n239 = Copy(10:w423, 11:w422) -> ()  [unwired: 1 in, 5 out]
            }
            frame True {
            }
          }
        }
        n240 = call "Create_directory_path.vi"("Path name"=w400) -> ("Path name Out"=w399:path)
        n241 = Move(source path=w406, 10:w399) -> ()  [unwired: 1 in, 5 out]
      }
      frame "Install Adam setup files" {
        w427 = "Current_Setup.xls"
        n242 = global read "Constants_global.vi" "ADAM setups folder"() -> (w429:path)
        n243 = Build Path(base path=w429, name or relative path="Setup_Files") -> (appended path=w426:path)
        n244 = Build Path(base path=w426, name or relative path=w427) -> (appended path=w424:path)
        n245 = call "Does_file_exist_(simple).vi"("Pathname"=w424) -> ("exists?"=w425:bool)
        n246 = case shown="False" w425 {
          tunnel: w424 -> [w440 _]
          tunnel: w427 -> [w438 _]
          frame False {
            n247 = local read "Templates"() -> (w439:path)
            n248 = Build Path(base path=w439, name or relative path="ADAM_Setup_files") -> (appended path=w437:path)
            n249 = Build Path(base path=w437, name or relative path=w438) -> (appended path=w436:path)
            n250 = Copy(10:w440, 11:w436) -> ()  [unwired: 1 in, 5 out]
          }
          frame True {
          }
        }
        n251 = Build Array (concatenate)(w431, w424) -> (w430:path[])
      }
      frame "Choose ADAM Setup file" {
        w449 = "Selected_Filename.txt" ("Substring")
        n252 = global read "Constants_global.vi" "ADAM setups folder"() -> (w453:path)
        n253 = Build Path(base path=w453, name or relative path="Setup_Files") -> (appended path=w450:path)
        n254 = Build Path(base path=w450, name or relative path=w449) -> (appended path=w448:path)
        n255 = call "Read_File_Simple.vi"("Filename"=w448) -> ("string"=w446:string)  [unwired: 2 in, 7 out]
        n256 = Build Array(w449) -> (w451:string[])
        n257 = call "List_files_in_order_of_age.vi"("Files to Hide"=w451, "Folder"=w450) -> ("file names"=w447:string[])
        n258 = Search 1D Array(1D array=w447, element=w446) -> (index of element=w443:i32)  [unwired: 1 out]
        n259 = property on="ADAM Setup File" class="Ring (strict)"("Strings []"=w447) -> ()  [unwired: 2 in, 2 out]
        n260 = Less Than 0?(x=w443) -> (x < 0?=w444:bool)
        n261 = Select(t=0, s=w444, f=w443) -> (s? t:f=w442:i32)
        n262 = local write "ADAM Setup File"(w442) -> ()
      }
      frame "Preference files continued" {
        n263 = global read "Constants_global.vi" "Calib setups folder"() -> (w465:path)
        n264 = Build Array("Hot_Wire_Bridges.txt", "Hot_Wire_Probes.txt", "Pressure_Transducers.txt") -> (w460:string[])
        n265 = for {
          tunnel: w460 -> [w469] mode=indexing
          tunnel: w465 -> [w470]
          tunnel: [w468] -> w458 mode=indexing
          n266 = Build Path(base path=w470, name or relative path=w469) -> (appended path=w468:path)
          n267 = call "Does_file_exist_(simple).vi"("Pathname"=w468) -> ("exists?"=w471:bool)
          n268 = case shown="False" w471 {
            tunnel: w468 -> [w475 _]
            tunnel: w469 -> [w472 _]
            frame False {
              n269 = local read "Templates"() -> (w473:path)
              n270 = Build Path(base path=w473, name or relative path=w472) -> (appended path=w474:path)
              n271 = Copy(10:w475, 11:w474) -> ()  [unwired: 1 in, 5 out]
            }
            frame True {
            }
          }
        }
        n272 = Build Array (concatenate)(w459, w458) -> (w457:path[])
      }
      frame "Variable Names" {
        n273 = Build Array("PWA Device Serial No.", "Analogue Device Serial No.", "Server address", "Server port number", "LabVIEW Administrators", "SMTP server IP address", "Server Comms", "Default Source Establishment Time (s)", "Temperature", "Abs Press (mbar)", "Default Traverse Name", "Tunnel Speed Control", "Current Overhead Factor", "Qnet Site Root", "Auto Calib Error fr Previous", "Auto Calib Error fr First") -> (w492:string[])
        n274 = case shown="\"Load, Edit then Save\"" w486 {
          tunnel: ["Load From Preference file" w498 "Save Preference File"] -> w487
          frame "Load Preferences from file" {
          }
          frame "Load, Edit then Save" {
            n275 = local read "OK"() -> (w501:bool)
            n276 = Select(t="Save Preference File", s=w501, f="Load From Preference file") -> (s? t:f=w498:string)
          }
          frame "Save Preferences to file" {
          }
        }
      }
      frame "Load From Preference file" {
        n277 = global read "Constants_global.vi" "General folder"() -> (w511:path)
        n278 = Build Path(base path=w511, name or relative path=w510) -> (appended path=w507:path)
        n279 = call "Read_File_Simple.vi"("Filename"=w507) -> ("string"=w512:string)  [unwired: 2 in, 7 out]
        n280 = for {
          tunnel: w514 -> [w517] mode=indexing
          tunnel: w512 -> [w516]
          w519 = FALSE  # Show Dialog?
          n281 = call "Get_Characters_from_string.vi"("Show Dialog?"=w519, "Input string"=w516, "Variable name"=w517) -> ("Status"=w518:enum16{"Char in string", "Char not in string"}, "Value"=w515:string)
          n282 = case shown="\"Char in string\"" w518 {
            tunnel: w517 -> [w521 _]
            tunnel: w515 -> [w520 _]
            frame "Char in string" {
              n283 = case shown="\"Server address\"" w521 {
                tunnel: w521 -> [w523 _ _ _ _ _ _ _ _ _ _ _ _ _ _ _ _]
                tunnel: w520 -> [_ w524 w525 w528 w529 w530 w532 w534 w537 _ w541 w545 w546 w548 w550 w553 w555]
                tunnel: w520 -> [_ _ _ _ _ _ _ _ _ w538 _ _ _ _ _ _ _]
                frame "No Match", Default {
                  n284 = call "Was_string_matched.vi"("Match Error"=TRUE, "Variable name"=w523) -> ()  [unwired: 1 in]
                }
                frame "Server address" {
                  n285 = global write "Preference_global.vi" "Server address"(w524) -> ()
                  n286 = local write "Server address"(w524) -> ()
                }
                frame "Default Traverse Name" {
                  n287 = global write "Trav_pos_global.vi" "Default Traverse Setup"(w525) -> ()
                }
                frame "Server port number" {
                  n288 = Decimal String To Number(string=w528) -> (number=w527:i32)  [unwired: 3 out]
                  n289 = To Unsigned Long Integer(number=w527) -> (unsigned 32bit integer=w526:u32)
                  n290 = local write "Server port number"(w526) -> ()
                  n291 = global write "Preference_global.vi" "Server port number"(w526) -> ()
                }
                frame "Analogue Device Serial No." {
                  n292 = local write "Analogue Device Serial No."(w529) -> ()
                }
                frame "PWA Device Serial No." {
                  n293 = local write "PWA Device Serial No."(w530) -> ()
                }
                frame "Default Source Establishment Time (s)" {
                  n294 = Fract/Exp String To Number(string=w532) -> (number=w531:dbl)  [unwired: 4 out]
                  n295 = global write "Preference_global.vi" "Default Source Establishment Time (s)"(w531) -> ()
                  n296 = local write "Default Source Establishment Time (s)"(w531) -> ()
                }
                frame "Tunnel Speed Control" {
                  n297 = Equal?(x="TRUE", y=w534) -> (x = y?=w533:bool)
                  n298 = local write "Tunnel Speed Control"(w533) -> ()
                  n299 = global write "Preference_global.vi" "Tunnel Speed Control"(w533) -> ()
                }
                frame "LabVIEW Administrators" {
                  n300 = call "Get_array_values_fr_String.vi"("String Value"=w537) -> ("String array"=w536:string[])  [unwired: 1 out]
                  n301 = global write "Preference_global.vi" "LabVIEW Administrators"(w536) -> ()
                  n302 = local write "LabVIEW Administrators"(w536) -> ()
                }
                frame "SMTP server IP address" {
                  n303 = local write "SMTP server IP address"(w538) -> ()
                  n304 = global write "Preference_global.vi" "SMTP server IP address"(w538) -> ()
                }
                frame "Server Comms" {
                  n305 = Equal?(x="TRUE", y=w541) -> (x = y?=w540:bool)
                  n306 = case shown="False" w540 {
                    tunnel: [Server_Comms."Do Not Link To Server" ("Server Comms") Server_Comms."Server Link Healthy" ("Server Comms")] -> w539
                    frame False {
                    }
                    frame True {
                    }
                  }
                  n307 = local write "Server Comms"(w539) -> ()
                  n308 = global write "Preference_global.vi" "Server Comms"(w539) -> ()
                }
                frame "Temperature" {
                  n309 = global write "Preference_global.vi" "Temperature"(w545) -> ()
                  n310 = local write "Temperature"(w545) -> ()
                }
                frame "Abs Press (mbar)" {
                  n311 = global write "Preference_global.vi" "Abs Press (mbar)"(w546) -> ()
                  n312 = local write "Abs Press (mbar)"(w546) -> ()
                }
                frame "Qnet Site Root" {
                  n313 = String To Path(string=w548) -> (path=w547:path)
                  n314 = global write "Qnet_Globals.vi" "Local Site Root"(w547) -> ()
                  n315 = local write "Qnet Site Root"(w547) -> ()
                }
                frame "Current Overhead Factor" {
                  n316 = Fract/Exp String To Number(string=w550) -> (number=w549:dbl)  [unwired: 4 out]
                  n317 = call "Overhead_Factor.vi"("Current Overhead Factor In"=w549, "Mode"=Overhead."Initialise totals to 3hr") -> ()  [unwired: 2 in, 1 out]
                }
                frame "Auto Calib Error fr Previous" {
                  n318 = Fract/Exp String To Number(string=w553) -> (number=w552:dbl)  [unwired: 4 out]
                  n319 = global write "Preference_global.vi" "% Error From Previous Calib"(w552) -> ()
                  n320 = local write "% Error From Previous Calib"(w552) -> ()
                }
                frame "Auto Calib Error fr First" {
                  n321 = Fract/Exp String To Number(string=w555) -> (number=w554:dbl)  [unwired: 4 out]
                  n322 = global write "Preference_global.vi" "% Error From First Calib"(w554) -> ()
                  n323 = local write "% Error From First Calib"(w554) -> ()
                }
              }
            }
            frame "Char not in string" {
            }
          }
        }
        n324 = local read "Post Processing Machine"() -> (w506:bool)
        n325 = Select(t="Check file permission status", s=w506, f="is traverse setup blank?") -> (s? t:f=w504:string)
        n326 = Build Array (concatenate)(w509, w507) -> (w508:path[])
      }
      frame "is traverse setup blank?" {
        n327 = local read "Data Folder"() -> (w562:path)
        n328 = global read "Trav_pos_global.vi" "Default Traverse Setup"() -> (w556:string)
        n329 = Build Path(base path=w562, name or relative path="Preferences") -> (appended path=w561:path)
        n330 = Build Path(base path=w561, name or relative path=w565) -> (appended path=w560:path)
        n331 = List Folder(path=w560) -> (folder names=w558:string[])  [unwired: 1 in, 5 out]
        n332 = Search 1D Array(1D array=w558, element=w556) -> (index of element=w559:i32)  [unwired: 1 out]
        n333 = case shown="0, Default" w559 {
          tunnel: w558 -> [_ w571]
          tunnel: [w569 w570] -> w557
          tunnel: w556 -> [w569 _]
          frame 0, Default {
          }
          frame -1 {
            n334 = Index Array(array=w571, index=0) -> (element=w570:string)
          }
        }
        n335 = global write "Trav_pos_global.vi" "Default Traverse Setup"(w557) -> ()
      }
      frame "Please Enter new  Traverse Setup" {
        n336 = global read "Trav_pos_global.vi" "Default Traverse Setup"() -> (w575:string)
        n337 = String Length(string=w575) -> (length=w580:i32)
        n338 = In Range and Coerce(upper limit=w577, x=w580, lower limit=w578) -> (In Range?=w576:bool)  [unwired: 1 out]
        n339 = case shown="False" w576 {
          tunnel: w575 -> [w591 w599]
          tunnel: ["Please Enter new  Traverse Setup" "Update Traverse setup menu ring"] -> w579
          tunnel: [w584 w599] -> w574
          tunnel: w578 -> [w588 _]
          tunnel: w577 -> [w587 _]
          frame False {
            n340 = Format Into String(format string="Please Enter a Traverse Setup Name\nIt must be between %d and %d Characters" ("Message to user"), w588, w587) -> (resulting string=w586:string)  [unwired: 2 in, 1 out]
            n341 = call "Input_String_Dialog.vi"("Value"=w591, "Message to user"=w586) -> ("Ok Out"=w583:bool, "Output string"=w585:string)
            n342 = case shown="False" w583 {
              tunnel: w585 -> [_ w596]
              tunnel: [w592 w595] -> w584
              frame False {
                n343 = property on="Default Traverse Name" class="Ring (strict)"() -> ("Strings []"=w593:string[])  [unwired: 2 in, 2 out]
                n344 = Index Array(array=w593, index=0) -> (element=w592:string)
              }
              frame True {
                n345 = call "Fast_string_Replace.vi"("Replace match with:"="_", "Input String"=w596, "regular expression"=" ") -> ("Output String"=w595:string)  [unwired: 2 out]
              }
            }
          }
          frame True {
          }
        }
        n346 = global write "Trav_pos_global.vi" "Default Traverse Setup"(w574) -> ()
      }
      frame "Update Traverse setup menu ring" {
        n347 = global read "Trav_pos_global.vi" "Default Traverse Setup"() -> (w604:string)
        n348 = local read "Data Folder"() -> (w610:path)
        n349 = Build Path(base path=w610, name or relative path="Preferences") -> (appended path=w609:path)
        n350 = Build Path(base path=w609, name or relative path=w602) -> (appended path=w608:path)
        n351 = List Folder(path=w608) -> (folder names=w606:string[])  [unwired: 1 in, 5 out]
        n352 = Build Array (concatenate)(w606, "--New Traverse Setup--") -> (w605:string[])
        n353 = Search 1D Array(1D array=w605, element=w604) -> (index of element=w612:i32)  [unwired: 1 out]
        n354 = case shown="-1" w612 {
          tunnel: [w618 0] -> w614
          tunnel: w605 -> [w617 w621]
          tunnel: w604 -> [_ w620]
          tunnel: w612 -> [w618 _]
          tunnel: [w617 w619] -> w603
          frame 0, Default {
          }
          frame -1 {
            n355 = Build Array (concatenate)(w620, w621) -> (w619:string[])
          }
        }
        n356 = local write "Default Traverse Name"(w614) -> ()
        n357 = property on="Default Traverse Name" class="Ring (strict)"("Strings []"=w603) -> ()  [unwired: 2 in, 2 out]
      }
      frame "Create Traverse setup" {
        n358 = local read "Templates"() -> (w624:path)
        n359 = Build Path(base path=w624, name or relative path="All_Traverses") -> (appended path=w630:path)
        n360 = stacked-sequence {
          seq-local: [w635 _] -> [_ w663]
          seq-local: [w634 _] -> [_ _]
          tunnel: w630 -> [w637 _]
          tunnel: [w640 _] -> w627
          tunnel: [w639 _] -> w626
          tunnel: w624 -> [_ w662]
          tunnel: [_ w660] -> w623
          frame #0 {
            w643 = "Default_Space_file.xls" ("name or relative path")
            w638 = "Traverse_Setup.xls" ("name or relative path")
            n361 = global read "Trav_pos_global.vi" "Default Traverse Setup"() -> (w634:string)
            n362 = global read "Constants_global.vi" "Traverse folder"() -> (w647:path)
            n363 = Build Path(base path=w637, name or relative path=w643) -> (appended path=w641:path)
            n364 = Build Path(base path=w637, name or relative path=w638) -> (appended path=w636:path)
            n365 = Build Path(base path=w647, name or relative path=w634) -> (appended path=w635:path)
            n366 = Build Path(base path=w635, name or relative path="Trav_Space_Files") -> (appended path=w644:path)
            n367 = Build Path(base path=w644, name or relative path=w643) -> (appended path=w640:path)
            n368 = call "Does_file_exist_(simple).vi"("Pathname"=w640) -> ("exists?"=w642:bool)
            n369 = case shown="False" w642 {
              tunnel: w641 -> [w650 _]
              tunnel: w640 -> [w649 _]
              frame False {
                n370 = call "Create_directory_path.vi"("Path name"=w649) -> ("Path name Out"=w648:path)
                n371 = Copy(10:w648, 11:w650) -> ()  [unwired: 1 in, 5 out]
              }
              frame True {
              }
            }
            n372 = Build Path(base path=w635, name or relative path=w638) -> (appended path=w639:path)
            n373 = call "Does_file_exist_(simple).vi"("Pathname"=w639) -> ("exists?"=w646:bool)
            n374 = case shown="False" w646 {
              tunnel: w636 -> [w659 _]
              tunnel: w639 -> [w655 _]
              tunnel: w634 -> [w658 _]
              frame False {
                w651 = TRUE  # append to file? (new file:F)
                n375 = call "Create_directory_path.vi"("Path name"=w655) -> ("Path name Out"=w654:path)
                n376 = call "Read_File_Simple.vi"("Filename"=w659) -> ("string"=w657:string)  [unwired: 2 in, 7 out]
                n377 = call "Fast_string_Replace.vi"("Replace match with:"=w658, "Input String"=w657, "regular expression"="A_Tunnel") -> ("Output String"=w653:string)  [unwired: 2 out]
                n378 = call "Write_Characters_To_File.vi"("file path (dialog if empty)"=w654, "advisory dialog? (display:T)"=TRUE, "character string"=w653, "append to file? (new file:F)"=w651) -> ()  [unwired: 1 in, 4 out]
              }
              frame True {
              }
            }
          }
          frame #1 {
            w661 = "Traverse_Preferences.txt" ("name or relative path")
            n379 = Build Path(base path=w663, name or relative path=w661) -> (appended path=w660:path)
            n380 = Build Path(base path=w662, name or relative path=w661) -> (appended path=w664:path)
            n381 = call "Does_file_exist_(simple).vi"("Pathname"=w660) -> ("exists?"=w665:bool)
            n382 = case shown="False" w665 {
              tunnel: w664 -> [w668 _]
              tunnel: w660 -> [w667 _]
              frame False {
                n383 = call "Create_directory_path.vi"("Path name"=w667) -> ("Path name Out"=w666:path)
                n384 = Copy(10:w666, 11:w668) -> ()  [unwired: 1 in, 5 out]
              }
              frame True {
              }
            }
          }
        }
        n385 = Build Array (concatenate)(w629, w626, w623, w627) -> (w628:path[])
      }
      frame "Check file permission status" {
        n386 = for {
          tunnel: w673 -> [w687] mode=indexing
          shift-right: [w684] -> w670
          shift-left: "" -> [w685]
          n387 = call "Can_File_be_Editted.vi"("Filename"=w687) -> ("File Permissions OK?"=w688:bool, "Comment String"=w686:string)  [unwired: 2 out]
          n388 = case shown="False" w688 {
            tunnel: w687 -> [w693 _]
            tunnel: w686 -> [w692 _]
            tunnel: w685 -> [w691 w694]
            tunnel: [w690 w694] -> w684
            frame False {
              n389 = Format Into String(format string="\"%s\" %s\n", initial string=w691, w693, w692) -> (resulting string=w690:string)  [unwired: 1 in, 1 out]
            }
            frame True {
            }
          }
        }
        n390 = case shown="\"Load, Edit then Save\"" w674 {
          tunnel: ["Output Dev Number" w696 "Output Dev Number"] -> w675
          frame "Save Preferences to file" {
          }
          frame "Load, Edit then Save" {
            n391 = local read "Post Processing Machine"() -> (w699:bool)
            n392 = Select(t="Data Folder Changed?", s=w699, f="What next1") -> (s? t:f=w696:string)
          }
          frame "Load Preferences from file" {
          }
        }
        n393 = Empty String/Path?(string/path=w670) -> (empty?=w671:bool)
        n394 = case shown="True" w671 {
          tunnel: w670 -> [w683 _]
          frame False {
            n395 = Concatenate Strings("The following file permissions need to be sorted out before the software will run correctly.\n\n" ("string"), w683) -> (w681:string)
            n396 = Two Button Dialog(message=w681, 1:"Continue" ("F button name (\"Cancel\")"), 2:"Abort" ("F button name (\"Cancel\")")) -> (T button?=w678:bool)
            n397 = Stop(stop? (T)=w678) -> ()
          }
          frame True {
          }
        }
      }
      frame "What next1" {
        n398 = property on="Rig Setup" class="Ring (strict)"() -> ("Strings []"=w703:string[])  [unwired: 2 in, 2 out]
        n399 = Array Size(array=w703) -> (size(s)=w707:i32)
        n400 = Decrement(x=w707) -> (x-1=w706:i32)
        n401 = Equal?(x=w706, y="Rig Setup") -> (x = y?=w705:bool)
        n402 = case shown="False" w705 {
          tunnel: [w711 "Please Enter New Rig Name" ("t")] -> w704
          tunnel: w703 -> [w714 _]
          tunnel: "Rig Setup" -> [w713 _]
          frame False {
            n403 = global read "Preference_global.vi" "Rig Setup"() -> (w715:string)
            n404 = Index Array(array=w714, index=w713) -> (element=w710:string)
            n405 = Not Equal?(x=w710, y=w715) -> (x != y?=w712:bool)
            n406 = case shown="False" w712 {
              tunnel: ["What next2" ("f") "Update Rig setup menu ring" ("t")] -> w711
              tunnel: w710 -> [_ w717]
              frame False {
              }
              frame True {
                n407 = global write "Preference_global.vi" "Rig Setup"(w717) -> ()
              }
            }
          }
          frame True {
            n408 = global write "Preference_global.vi" "Rig Setup"("") -> ()
          }
        }
      }
      frame "What next2" {
        n409 = property on="Default Traverse Name" class="Ring (strict)"() -> ("Strings []"=w723:string[])  [unwired: 2 in, 2 out]
        n410 = Array Size(array=w723) -> (size(s)=w727:i32)
        n411 = Decrement(x=w727) -> (x-1=w726:i32)
        n412 = Equal?(x=w726, y="Default Traverse Name") -> (x = y?=w725:bool)
        n413 = case shown="False" w725 {
          tunnel: [w731 "Please Enter new  Traverse Setup" ("t")] -> w724
          tunnel: w723 -> [w735 _]
          tunnel: "Default Traverse Name" -> [w734 _]
          frame False {
            n414 = global read "Trav_pos_global.vi" "Default Traverse Setup"() -> (w733:string)
            n415 = Index Array(array=w735, index=w734) -> (element=w730:string)
            n416 = Not Equal?(x=w730, y=w733) -> (x != y?=w732:bool)
            n417 = case shown="False" w732 {
              tunnel: ["Data Folder Changed?" ("f") "Update Traverse setup menu ring" ("t")] -> w731
              tunnel: w730 -> [_ w737]
              frame False {
              }
              frame True {
                n418 = global write "Trav_pos_global.vi" "Default Traverse Setup"(w737) -> ()
              }
            }
          }
          frame True {
            n419 = global write "Trav_pos_global.vi" "Default Traverse Setup"("") -> ()
          }
        }
      }
      frame "Data Folder Changed?" {
        w742 = "Please Select your data folder"
        n420 = global read "Constants_global.vi" "Data Folder"() -> (w749:path)
        n421 = local read "Data Folder"() -> (w750:path)
        n422 = property on="OK" class="Bool (strict)"("Visible"=TRUE) -> ()  [unwired: 2 in, 2 out]
        n423 = while {
          shift-right: [w759] -> _
          shift-left: _ -> [w758]
          tunnel: [w757] -> w744
          stop <- TRUE stop-if-true
          n424 = local read "Post Processing Machine"() -> (w759:bool)
          n425 = Not Equal?(x=w759, y=w758) -> (x != y?=w757:bool)
        }
        n426 = Not Equal?(x=w749, y=w750) -> (x != y?=w748:bool)
        n427 = Select(t=w742, s=w748, f="Has OK has been pressed?") -> (s? t:f=w741:string)
        n428 = case shown="True" w744 {
          tunnel: [w753 w755] -> w743
          tunnel: w742 -> [_ w755]
          tunnel: w741 -> [w753 _]
          frame False {
          }
          frame True {
            n429 = global write "Preference_global.vi" "Rig Setup"("") -> ()
          }
        }
      }
      frame "Has OK has been pressed?" {
        n430 = flat-sequence {
          tunnel: ["OK"] -> w761
          frame #0 {
            n431 = Wait (ms)(milliseconds to wait=u32 100) -> ()  [unwired: 1 out]
          }
          frame #1 {
          }
        }
        n432 = local read "Post Processing Machine"() -> (w762:bool)
        n433 = case shown="False" w761 {
          tunnel: w762 -> [w767 w773]
          tunnel: [w766 w770] -> w760
          frame False {
            n434 = Select(t="Data Folder Changed?", s=w767, f="What next1") -> (s? t:f=w766:string)
          }
          frame True {
            n435 = Select(t="Save Preference File", s=w773, f="Output Dev Number") -> (s? t:f=w770:string)
          }
        }
      }
      frame "Output Dev Number" {
        n436 = stacked-sequence {
          seq-local: [w781 _ _] -> [_ w817 _]
          tunnel: w778 -> [_ _ _]
          frame #0 {
            w784 = T8 0 items=["Canonical Names Only"=0, "Aliases Only"=1, "Include Matching Aliases"=2, "Include All Aliases"=4] ("Search Mode")
            n437 = VISA Find Resource(10:w784) -> (3:w783:string[])  [unwired: 1 in, 3 out]
            n438 = for {
              shift-right: [w799] -> w781
              shift-left: string[] [] -> [w800]
              tunnel: w783 -> [w789] mode=indexing
              n439 = Reverse String(1:w789) -> (0:w797:string)
              n440 = Match Pattern(string=w797, regular expression="::") -> (before substring=w796:string)  [unwired: 4 out]
              n441 = Match Pattern(string=w789, regular expression="NI-VISA") -> (offset past match=w788:i32)  [unwired: 4 out]
              n442 = Reverse String(1:w796) -> (0:w794:string)
              n443 = Less Than 0?(x=w788) -> (x < 0?=w786:bool)
              n444 = Equal?(x=w794, y="INSTR") -> (x = y?=w792:bool)
              n445 = Equal?(x=w794, y="RAW") -> (x = y?=w791:bool)
              n446 = Or(x=w792, y=w791) -> (x .or. y?=w787:bool)
              n447 = And(x=w787, y=w786) -> (x .and. y?=w785:bool)
              n448 = case shown="True" w785 {
                tunnel: w800 -> [w801 w804]
                tunnel: [w801 w803] -> w799
                tunnel: w789 -> [_ w802]
                frame False {
                }
                frame True {
                  n449 = Build Array (concatenate)(w804, w802) -> (w803:string[])
                }
              }
            }
          }
          frame #1 {
            w809 = "Dev" ("format string")
            n450 = local read "Analogue Device Serial No."() -> (w813:string)
            n451 = String Length(string=w809) -> (length=w811:i32)
            n452 = local read "PWA Device Serial No."() -> (w807:string)
            n453 = String Subset(string=w813, length (rest)=w811) -> (substring=w815:string)  [unwired: 1 out]
            n454 = String Subset(string=w807, length (rest)=w811) -> (substring=w810:string)  [unwired: 1 out]
            n455 = Equal?(x=w815, y=w809) -> (x = y?=w812:bool)
            n456 = Equal?(x=w809, y=w810) -> (x = y?=w808:bool)
            n457 = for {
              tunnel: w813 -> [w836]
              tunnel: w817 -> [w834] mode=indexing
              tunnel: [w835] -> w829 mode=indexing
              tunnel: w807 -> [w833]
              tunnel: [w832] -> w826 mode=indexing
              n458 = Match Pattern(string=w834, regular expression=w836) -> (offset past match=w835:i32)  [unwired: 1 in, 3 out]
              n459 = Match Pattern(string=w834, regular expression=w833) -> (offset past match=w832:i32)  [unwired: 1 in, 3 out]
            }
            n460 = Array Max & Min(array=w829) -> (max index (indices)=w830:i32)  [unwired: 3 out]
            n461 = Array Max & Min(array=w826) -> (max index (indices)=w828:i32)  [unwired: 3 out]
            n462 = Increment(x=w828) -> (x+1=w819:i32)
            n463 = Increment(x=w830) -> (x+1=w823:i32)
            n464 = Equal To 0?(x=w823) -> (x = 0?=w825:bool)
            n465 = Equal To 0?(x=w819) -> (x = 0?=w820:bool)
            n466 = Select(t=1, s=w825, f=w823) -> (s? t:f=w824:i32)
            n467 = Select(t=1, s=w820, f=w819) -> (s? t:f=w818:i32)
            n468 = Format Into String(format string="Dev%d", w824) -> (resulting string=w814:string)  [unwired: 2 in, 1 out]
            n469 = Format Into String(format string="Dev%d", w818) -> (resulting string=w806:string)  [unwired: 2 in, 1 out]
            n470 = Select(t=w813, s=w812, f=w814) -> (s? t:f=w816:string)
            n471 = Select(t=w807, s=w808, f=w806) -> (s? t:f=w805:string)
            n472 = global write "PWAtasksGLOBAL.vi" "Analogue Dev Name"(w816) -> ()
            n473 = global write "PWAtasksGLOBAL.vi" "PWA Dev Name"(w805) -> ()
          }
          frame #2 {
            n474 = for {
              tunnel: string[] ["Raw_Calibrations", "Raw_Measurements", "Results", "Calibrations", "Commands"] -> [w841] mode=indexing
              n475 = call "Data_folder_Path.vi"("Data Type"=w841) -> ("Data Folder"=w840:path)  [unwired: 1 in]
              n476 = Build Path(base path=w840, name or relative path="Test" ("Substring")) -> (appended path=w843:path)
              n477 = call "Create_directory_path.vi"("Path name"=w843) -> ()  [unwired: 1 out]
            }
            n478 = call "Data_folder_Path.vi"("Data Type"="Results_Post_Processed" ("element")) -> ("Data Folder"=w837:path)  [unwired: 1 in]
            n479 = call "Create_directory_path.vi"("Path name"=w837) -> ()  [unwired: 1 out]
          }
        }
      }
      frame "Save Preference File" {
        n480 = global read "Constants_global.vi" "General folder"() -> (w847:path)
        n481 = call "Date_and_Time_to_string.vi"() -> ("Date and time (spreadsheet)"=w855:string)
        n482 = Build Path(base path=w847, name or relative path=w846) -> (appended path=w845:path)
        n483 = for {
          tunnel: w854 -> [w865] mode=indexing
          shift-right: [w861] -> w853
          shift-left: w855 -> [w863]
          n484 = case shown="\"Analogue Device Serial No.\"" w865 {
            tunnel: w865 -> [w868 _ _ _ _ _ _ _ _ _ _ _ _ _ _ _ _]
            tunnel: ["No Match" "Server address" w871 w873 w875 w879 "SMTP server IP address" "PWA Device Serial No." "Analogue Device Serial No." w883 w885 "Temperature" "Abs Press (mbar)" w890 w895 w898 w901] -> w864
            frame "No Match", Default {
              n485 = call "Was_string_matched.vi"("Match Error"=TRUE, "Variable name"=w868) -> ()  [unwired: 1 in]
            }
            frame "Server address" {
              n486 = global write "Preference_global.vi" "Server address"("Server address") -> ()
            }
            frame "Server port number" {
              n487 = global write "Preference_global.vi" "Server port number"("Server port number") -> ()
              n488 = Number To Decimal String(number="Server port number") -> (decimal integer string=w871:string)  [unwired: 1 out]
            }
            frame "Default Source Establishment Time (s)" {
              n489 = global write "Preference_global.vi" "Default Source Establishment Time (s)"("Default Source Establishment Time (s)") -> ()
              n490 = Number To Decimal String(number="Default Source Establishment Time (s)") -> (decimal integer string=w873:string)  [unwired: 1 out]
            }
            frame "Tunnel Speed Control" {
              n491 = global write "Preference_global.vi" "Tunnel Speed Control"("Tunnel Speed Control") -> ()
              n492 = Select(t="TRUE", s="Tunnel Speed Control", f="FALSE") -> (s? t:f=w875:string)
            }
            frame "LabVIEW Administrators" {
              n493 = global write "Preference_global.vi" "LabVIEW Administrators"("LabVIEW Administrators") -> ()
              n494 = call "Put_Array_into_String.vi"("String array"="LabVIEW Administrators") -> ("String Value"=w879:string)
            }
            frame "SMTP server IP address" {
              n495 = global write "Preference_global.vi" "SMTP server IP address"("SMTP server IP address") -> ()
            }
            frame "PWA Device Serial No." {
            }
            frame "Analogue Device Serial No." {
            }
            frame "Default Traverse Name" {
              n496 = global read "Trav_pos_global.vi" "Default Traverse Setup"() -> (w883:string)
            }
            frame "Server Comms" {
              n497 = case shown="\"Server Link Healthy\"" "Server Comms" {
                tunnel: ["TRUE" "FALSE"] -> w885
                frame "Server Link Healthy" {
                }
                frame "Do Not Link To Server" {
                }
              }
              n498 = global write "Preference_global.vi" "Server Comms"("Server Comms") -> ()
            }
            frame "Temperature" {
              n499 = global write "Preference_global.vi" "Temperature"("Temperature") -> ()
            }
            frame "Abs Press (mbar)" {
              n500 = global write "Preference_global.vi" "Abs Press (mbar)"("Abs Press (mbar)") -> ()
            }
            frame "Current Overhead Factor" {
              n501 = call "Overhead_Factor.vi"("Mode"=Overhead."Read Current Overhead") -> ("Current Overhead Factor"=w892:dbl)  [unwired: 3 in]
              n502 = Number To Fractional String(number=w892, precision (6)=i16 4) -> (F-format string=w890:string)  [unwired: 2 out]
            }
            frame "Auto Calib Error fr Previous" {
              n503 = global write "Preference_global.vi" "% Error From Previous Calib"("% Error From Previous Calib") -> ()
              n504 = Number To Fractional String(number="% Error From Previous Calib", precision (6)=i16 2) -> (F-format string=w895:string)  [unwired: 2 out]
            }
            frame "Auto Calib Error fr First" {
              n505 = global write "Preference_global.vi" "% Error From First Calib"("% Error From First Calib") -> ()
              n506 = Number To Fractional String(number="% Error From First Calib", precision (6)=i16 2) -> (F-format string=w898:string)  [unwired: 2 out]
            }
            frame "Qnet Site Root" {
              n507 = global write "Qnet_Globals.vi" "Local Site Root"("Qnet Site Root") -> ()
              n508 = Path To String(path="Qnet Site Root") -> (string=w901:string)
            }
          }
          n509 = call "Characters_to_string.vi"("Characters to write"=w864, "Label for characters"=w865) -> ("Output string"=w862:string)
          n510 = Concatenate Strings(w863, w862) -> (w861:string)
        }
        n511 = case shown="\"Load, Edit then Save\"" w849 {
          tunnel: [TRUE TRUE TRUE] -> w848
          frame "Load, Edit then Save" {
            n512 = Current VI's Path() -> (path=w857:path)
            n513 = call "Open_Close_Front_Panel.ph.vi"("Front Panel Window:Open"=FALSE, "VI path"=w857) -> ()  [unwired: 2 out]
          }
          frame "Load Preferences from file" {
          }
          frame "Save Preferences to file" {
          }
        }
        n514 = call "Write_Characters_To_File.vi"("file path (dialog if empty)"=w845, "advisory dialog? (display:T)"=FALSE, "character string"=w853, "append to file? (new file:F)"=FALSE) -> ()  [unwired: 1 in, 4 out]
      }
      frame "Save SW Preferences" {
        w917 = FALSE  # append to file? (new file:F)
        w918 = FALSE  # advisory dialog? (display:T)
        n515 = local read "Post Processing Machine"() -> (w907:bool)
        n516 = Path To String(path="Data Folder") -> (string=w909:string)
        n517 = global read "Preference_global.vi" "Server Comms"() -> (w913:T2)
        n518 = call "Characters_to_string.vi"("Characters to write"=w909, "Label for characters"=w911) -> ("Output string"=w919:string)
        n519 = Select(t="True", s=w907, f="False") -> (s? t:f=w904:string)
        n520 = call "Characters_to_string.vi"("Characters to write"=w904, "Label for characters"=w902) -> ("Output string"=w903:string)
        n521 = call "Date_and_Time_to_string.vi"() -> ("Date and time (spreadsheet)"=w914:string)
        n522 = case shown="\"Server Link Healthy\"" w913 {
          tunnel: ["Update Served VI file" "Update Local Adam Table"] -> w912
          frame "Server Link Healthy" {
          }
          frame "Do Not Link To Server" {
          }
        }
        n523 = Concatenate Strings(w914, w919, w903) -> (w915:string)
        n524 = local read "EnFlo SW Preferences"() -> (w916:path)
        n525 = call "Write_Characters_To_File.vi"("file path (dialog if empty)"=w916, "advisory dialog? (display:T)"=w918, "character string"=w915, "append to file? (new file:F)"=w917) -> ()  [unwired: 1 in, 4 out]
      }
      frame "Update Local Adam Table" {
        n526 = stacked-sequence {
          seq-local: [w933 _] -> [_ w947]
          tunnel: ["Update Served VI file" _] -> w925
          frame #0 {
            w933 = T9 {"Ch Name"="", "Type"=enum."4011", "Function"=enum."Analogue Input", "Ch State"=enum."On", "Calibration type"=enum."Raw", "A"=0.0, "B"=0.0, "C"=0.0, "D"=0.0, "Comments"="", "Address"={"Main"=0, "Ch."=0, "Sub"=0, "Port Name"=""}, "String"="", "Duty"=0} ("Ch Discription")
            n527 = global read "Preference_global.vi" "Abs Press (mbar)"() -> (w930:string)
            n528 = global read "Preference_global.vi" "Temperature"() -> (w931:string)
            n529 = Bundle By Name(cluster=w933, "Type"=Module_type_ADAM."Hold Value", "Calibration type"=Calib_type_ADAM."Raw", "A"=1.0) -> (w934:T9)
            n530 = Build Array(w931, w930) -> (w929:string[])
            n531 = for {
              tunnel: [w940] -> w932 mode=indexing
              tunnel: w934 -> [w939]
              tunnel: w929 -> [w938] mode=indexing
              n532 = Bundle By Name(cluster=w939, "Ch Name"=w938) -> (w940:T9)
            }
            n533 = call "Update_Ch_Discription_client.vi"("Channels to update In"=w932) -> ()  [unwired: 1 out]
          }
          frame #1 {
            n534 = global read "Preference_global.vi" "Rig Setup"() -> (w942:string)
            n535 = call "Get_Current_Scan_client.vi"() -> ("Ch Description Array"=w948:T9[])  [unwired: 1 in, 3 out]
            n536 = Match Pattern(string=w942, regular expression="-") -> (before substring=w941:string)  [unwired: 4 out]
            n537 = Format Into String(format string="%s Metadata:" ("Format String"), w941) -> (resulting string=w950:string)  [unwired: 2 in, 1 out]
            n538 = Initialize Array(w947, 0 ("dimension size")) -> (w945:T9[])
            n539 = for {
              shift-right: [w961] -> w944
              shift-left: w945 -> [w962]
              tunnel: w948 -> [w953] mode=indexing
              tunnel: w950 -> [w960]
              tunnel: "Metadata:" ("Format String") -> [w959]
              n540 = Unbundle By Name(w953) -> ("Ch Name"=w952:string)
              n541 = Match Pattern(string=w952, regular expression=w960) -> (offset past match=w957:i32)  [unwired: 4 out]
              n542 = Match Pattern(string=w952, regular expression=w959) -> (offset past match=w958:i32)  [unwired: 4 out]
              n543 = Greater Or Equal To 0?(x=w958) -> (x >= 0?=w955:bool)
              n544 = Less Than 0?(x=w957) -> (x < 0?=w956:bool)
              n545 = And(x=w956, y=w955) -> (x .and. y?=w954:bool)
              n546 = case shown="True" w954 {
                tunnel: w962 -> [w963 w968]
                tunnel: [w963 w967] -> w961
                tunnel: w953 -> [_ w966]
                frame False {
                }
                frame True {
                  n547 = Bundle By Name(cluster=w966, "Ch State"=Channel_State."Off") -> (w964:T9)
                  n548 = Build Array (concatenate)(w968, w964) -> (w967:T9[])
                }
              }
            }
            n549 = call "Update_Ch_Discription_client.vi"("Channels to update In"=w944) -> ()  [unwired: 1 out]
          }
        }
      }
      frame "Update Served VI file" {
        # "Template"
        # "Orig"
        n550 = global read "Constants_global.vi" "General folder"() -> (w977:path)
        n551 = Build Path(base path=w977, name or relative path=w970) -> (appended path=w972:path)
        n552 = Build Array("Served:VI:Name", "Served:VI:Path", "Server:IP Number:& Port No") -> (w974:string[])
        n553 = stacked-sequence {
          seq-local: [w980 _ _ _] -> [_ _ w990 _]
          seq-local: [_ w987 _ _] -> [_ _ w991 _]
          seq-local: [_ _ w992 _] -> [_ _ _ w1017]
          tunnel: w974 -> [w982 w988 _ w1018]
          tunnel: w972 -> [w981 _ _ w1019]
          tunnel: w970 -> [_ w984 _ _]
          frame #0 {
            n554 = call "Read_Ch_data_file.vi"("Present Channels"=w982, "Output"=enum16{"All Ch data", "The last few rows"}."All Ch data", "Filename"=w981) -> ("Channel Values"=w980:string[][])  [unwired: 2 in, 4 out]
          }
          frame #1 {
            n555 = local read "Templates"() -> (w986:path)
            n556 = Build Path(base path=w986, name or relative path=w984) -> (appended path=w985:path)
            n557 = call "Read_Ch_data_file.vi"("Present Channels"=w988, "Output"=enum16{"All Ch data", "The last few rows"}."All Ch data", "Filename"=w985) -> ("Channel Values"=w987:string[][])  [unwired: 2 in, 4 out]
          }
          frame #2 {
            n558 = Index Array(array=w990, index (col)=0 ("Index")) -> (element=w995:string[])  [unwired: 1 in]
            n559 = To Upper Case(1:w991) -> (0:w993:string[][])
            n560 = To Upper Case(1:w995) -> (0:w994:string[])
            n561 = for {
              tunnel: w994 -> [w998]
              tunnel: w991 -> [w1003] mode=indexing
              tunnel: w993 -> [w997] mode=indexing
              tunnel: [w1000] -> w992 mode=indexing
              tunnel: w990 -> [w999]
              n562 = Index Array(array=w997, index=0 ("Index")) -> (element=w1001:string)
              n563 = Search 1D Array(1D array=w998, element=w1001) -> (index of element=w1002:i32)  [unwired: 1 out]
              n564 = case shown="0, Default" w1002 {
                tunnel: w1003 -> [w1012 w1013]
                tunnel: w1002 -> [w1009 _]
                tunnel: [w1005 w1013] -> w1000
                tunnel: w999 -> [w1010 _]
                frame 0, Default {
                  n565 = Index Array(array=w1010, index (row)=w1009, index (col)=2 ("Index")) -> (element=w1007:string)
                  n566 = Array Subset(array=w1012, length=2) -> (w1006:string[])  [unwired: 1 in]
                  n567 = Build Array (concatenate)(w1006, w1007) -> (w1005:string[])
                }
                frame -1 {
                }
              }
            }
          }
          frame #3 {
            w1014 = FALSE  # Append last row only
            w1015 = FALSE  # Lock File
            w1016 = FALSE  # exists?
            n568 = call "Write_Ch_data_file.vi"("Append last row only"=w1014, "Lock File"=w1015, "exists?"=w1016, "Channel Values"=w1017, "Channel names"=w1018, "Filename"=w1019) -> ()  [unwired: 2 in, 4 out]
          }
        }
      }
      frame "Initialise Globals" {
        w1024 = TRUE  # OK
        w1028 = FALSE  # append to file? (new file:F)
        w1027 = FALSE  # advisory dialog? (display:T)
        n569 = global read "Constants_global.vi" "ADAM setups folder"() -> (w1034:path)
        n570 = global read "Constants_global.vi" "All_Users"() -> (w1023:path)
        n571 = property on="ADAM Setup File" class="Ring (strict)"() -> ("Strings []"=w1029:string[])  [unwired: 2 in, 2 out]
        n572 = Build Path(base path=w1023, name or relative path="Current_Username") -> (appended path=w1021:path)
        n573 = Build Path(base path=w1034, name or relative path="Setup_Files") -> (appended path=w1032:path)
        n574 = global read "Preference_global.vi" "User_Name"() -> (w1020:string)
        n575 = Build Path(base path=w1032, name or relative path="Selected_Filename.txt" ("Substring")) -> (appended path=w1025:path)
        n576 = call "Get_users_email_addresses.vi"("OK"=w1024) -> ()  [unwired: 5 out]
        n577 = Index Array(array=w1029, index="ADAM Setup File") -> (element=w1026:string)
        n578 = call "Write_File_Simple.vi"("character string"=w1020, "file path"=w1021) -> ()  [unwired: 1 in, 2 out]
        n579 = global write "Dynamic_call_global.ph.vi" "Acquisition Interlock"(FALSE ("Acquisition Interlock")) -> ()
        n580 = call "Write_Characters_To_File.vi"("file path (dialog if empty)"=w1025, "advisory dialog? (display:T)"=w1027, "character string"=w1026, "append to file? (new file:F)"=w1028) -> ()  [unwired: 1 in, 4 out]
      }
    }
  }
  n581 = call "Get_IP_Number.vi"() -> ("IP Number"=→"This Machine's IP Number":string)
